vi "Autonomous Independent.vi"() -> ()   [LabVIEW 2020]
doc: "This VI is called when autonomous begins, and will automatically be terminated when autonomous ends. You can carry out timed or sensor driven robot movement independently without needing to return to the caller."
uses:
  <vilib>/Rock Robotics/WPI/Solenoid/WPI_SolenoidValue.ctl
  <vilib>/Rock Robotics/WPI/ThirdParty/Phoenix-LabVIEW/Motor Controller/Controls/CTRE_Phoenix_MotorControl_ControlMode.ctl
  <vilib>/Rock Robotics/WPI/Utilities/WPI_GetSetVariantRefNum.vi
  <vilib>/Rock Robotics/WPI/Solenoid/WPI_SolenoidSetEnum.vi
  <vilib>/Rock Robotics/Network Tables/NT Read Number.vi
  GlobalDriveJoysticks.vi
  <vilib>/Rock Robotics/Network Tables/NT Read String.vi
  <vilib>/Rock Robotics/Network Tables/NT Write Numeric Array.vi
panel:
  out "Orange Limit Pressed 8":bool
  out "Blue Limit Pressed 8":bool
  out "Ty 8":dbl
  out "Orange Limit Pressed 7":bool
  out "Blue Limit Pressed 7":bool
  out "Ty 7":dbl
  out "Intake 4":bool
  out "Elevate 4":bool
  out "Orange Limit Pressed 6":bool
  out "Blue Limit Pressed 6":bool
  out "Ty 6":dbl
  out "Orange Limit Pressed 5":bool
  out "Blue Limit Pressed 5":bool
  out "Ty 5":dbl
  out "Intake 3":bool
  out "Elevate 3":bool
  out "Orange Limit Pressed 4":bool
  out "Blue Limit Pressed 4":bool
  out "Ty 4":dbl
  out "Orange Limit Pressed 3":bool
  out "Blue Limit Pressed 3":bool
  out "Ty 3":dbl
  out "Intake 2":bool
  out "Elevate 2":bool
  out "Orange Limit Pressed 2":bool
  out "Blue Limit Pressed 2":bool
  out "Ty 2":dbl
  out "Ty":dbl
  out "Blue Limit Pressed":bool
  out "Orange Limit Pressed":bool
  out "Elevate":bool
  out "Intake":bool
  # "Be sure to right-click and choose Data Operations>>Make Current Value default if you want to save the array values with the VI"
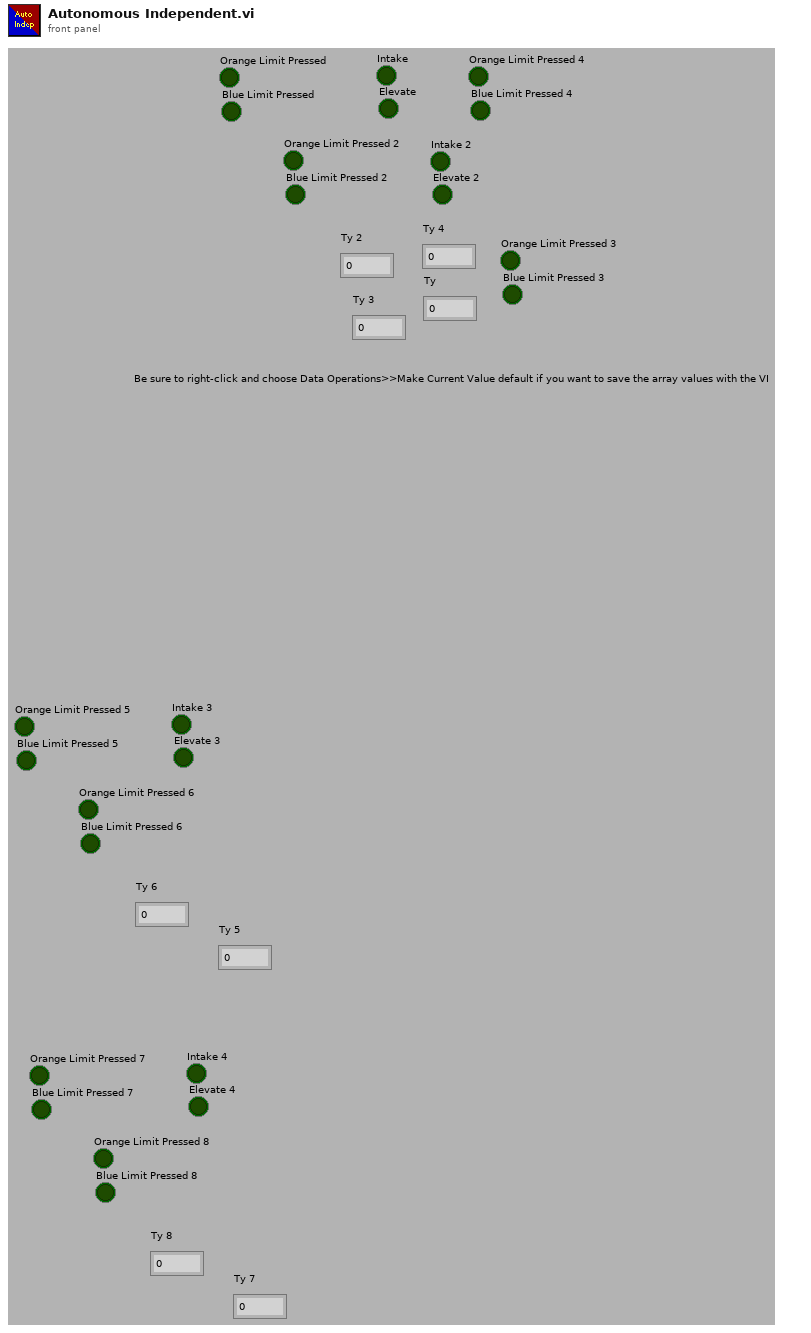
[diagram p1: front panel]
types:
  T1 = typedef "WPI_JoystickDevRef.ctl" = cluster{"Device":T2}
  T2 = typedef "WPI_JoystickDeviceEnum.ctl" = enum16{"USB 0", "USB 1", "USB 2", "USB 3", "USB 4", "USB 5"}
  T3 = typedef "WPI_SolenoidValue.ctl" = enum16{"Off", "On", "Forward", "Reverse"}
  T4 = typedef "WPI_SwitchDevRef.ctl" = cluster{"DevStatus":errorcluster, "DIO Channel":T5, "CntIndex":T6, "Normally Closed":bool}
  T5 = typedef "FPGA_DIOChannel.ctl" = enum8{"DIO 0", "DIO 1", "DIO 2", "DIO 3", "DIO 4", "DIO 5", "DIO 6", "DIO 7", "DIO 8", "DIO 9", "DIO MXP 0", "DIO MXP 1", "DIO MXP 2", "DIO MXP 3", "DIO MXP 4", "DIO MXP 5", "DIO MXP 6", "DIO MXP 7", "DIO MXP 8", "DIO MXP 9", "DIO MXP 10", "DIO MXP 11", "DIO MXP 12", "DIO MXP 13", "DIO MXP 14", "DIO MXP 15", "SPI Port CS1", "SPI Port CS2", "SPI Port CS3", "SPI Port MISO", "SPI Port MOSI", "Invalid"}
  T6 = typedef "FPGA_CounterCtrSystemIndex.ctl" = enum8{"Ctr 0", "Ctr 1", "Ctr 2", "Ctr 3", "Ctr 4", "Ctr 5", "Ctr 6", "Ctr 7", "Invalid"}
  T7 = typedef "WPI_SolenoidDevRef.ctl" = cluster{"DevStatus":errorcluster, "Pneumatics Control Module":u8, "Forward Solenoid Channel":T8, "Reverse Solenoid Channel":T8}
  T8 = typedef "WPI_SolenoidChannel.ctl" = enum8{"Solenoid 0", "Solenoid 1", "Solenoid 2", "Solenoid 3", "Solenoid 4", "Solenoid 5", "Solenoid 6", "Solenoid 7", "Solenoid 8", "Solenoid 9", "Solenoid 10", "Solenoid 11", "Solenoid 12", "Solenoid 13", "Solenoid 14", "Solenoid 15", "Invalid"}
  T9 = typedef "WPI_MotorControlDeviceRef.ctl" = cluster{"DeviceStatus":errorcluster, "Type":T10, "PWM":cluster{"PWM Channel":T11, "DeadBand":T12}, "CAN":cluster{"Device Number":u8, "SetOutput VI Ref":variant, "GetOutput VI Ref":variant, "Enable VI Ref":variant, "Disable VI Ref":variant, "Data":variant}, "Invert":bool, "DIO PWM":cluster{"PWM \"Enable\" Channel":T11, "DIOChannel":T5, "PWM Rate":dbl}}
  T10 = typedef "WPI_MotorControlType.ctl" = enum16{"PWM", "CAN", "DIO PWM"}
  T11 = typedef "FPGA_DIOPWMChannel.ctl" = enum8{"PWM 0", "PWM 1", "PWM 2", "PWM 3", "PWM 4", "PWM 5", "PWM 6", "PWM 7", "PWM 8", "PWM 9", "PWM MXP 0", "PWM MXP 1", "PWM MXP 2", "PWM MXP 3", "PWM MXP 4", "PWM MXP 5", "PWM MXP 6", "PWM MXP 7", "PWM MXP 8", "PWM MXP 9", "Invalid"}
  T12 = typedef "WPI_PWMDeadband.ctl" = cluster{"Name":string, "maxPositivePwm":i32, "minPositivePwm":i32, "centerPwm":i32, "maxNegativePwm":i32, "minNegativePwm":i32, "angularRange":u16}
  T13 = typedef "CTRE_Phoenix_MotorControl_ControlMode.ctl" = u16
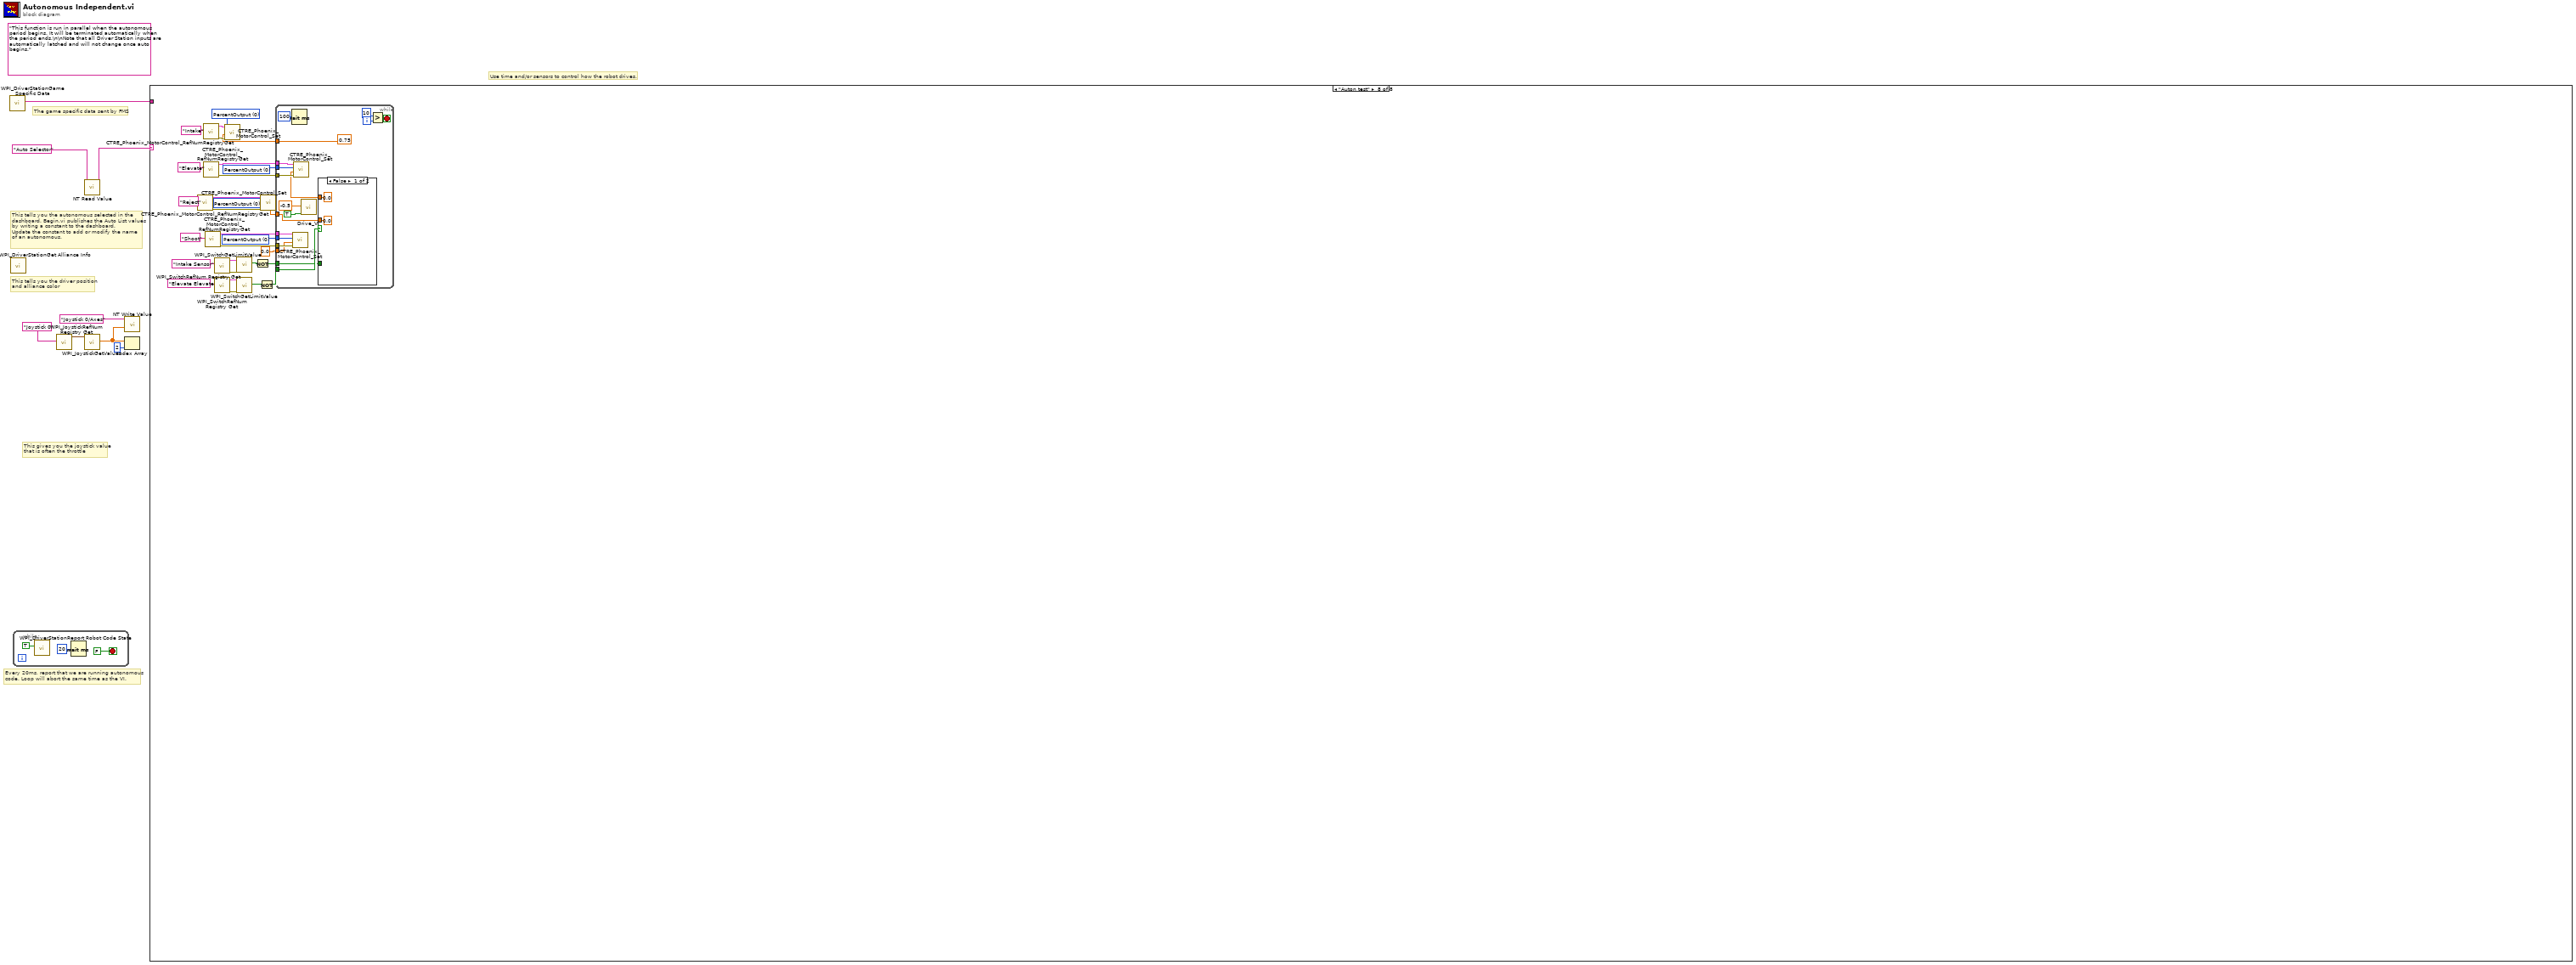
[diagram p0: block diagram]
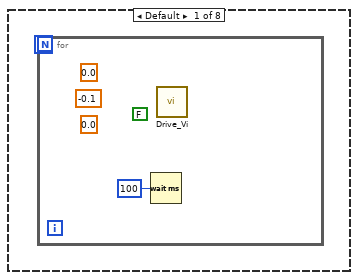
[diagram p2: hidden frame]
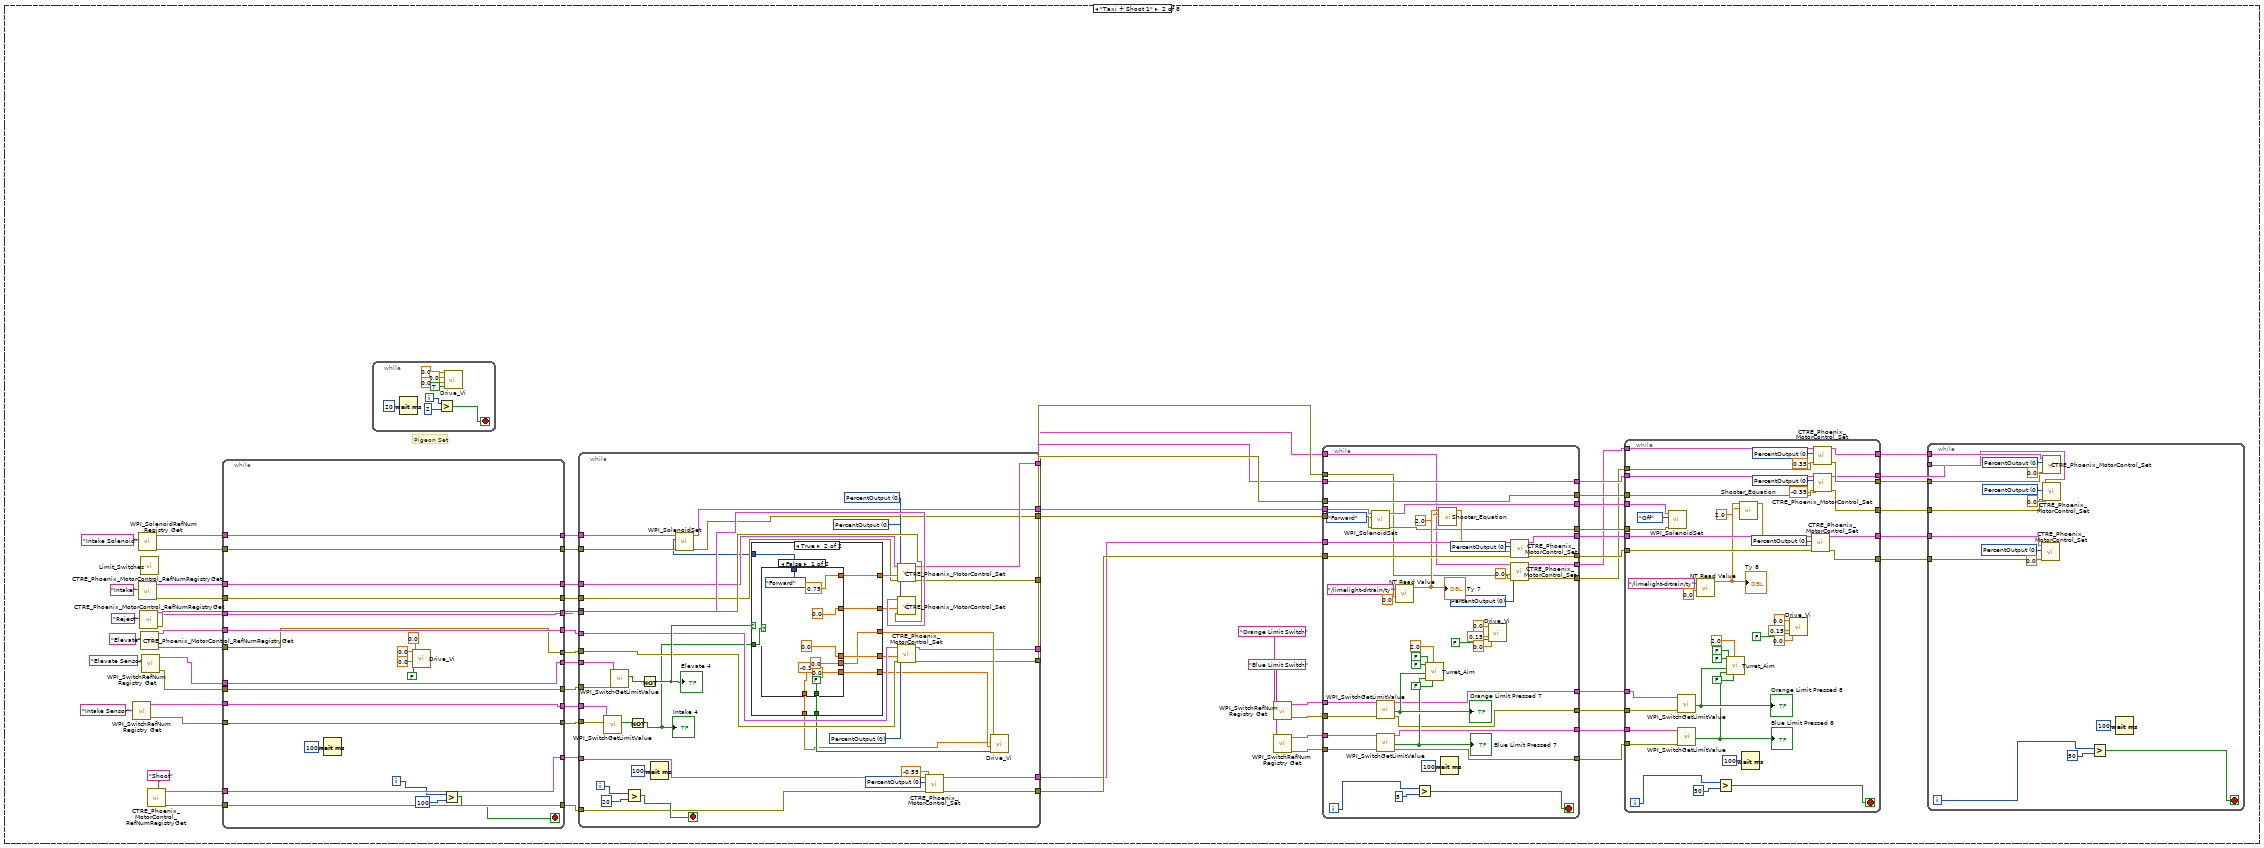
[diagram p3: hidden frame]
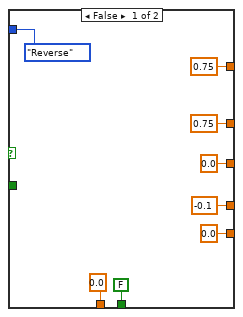
[diagram p4: hidden frame]
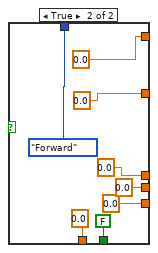
[diagram p5: hidden frame]
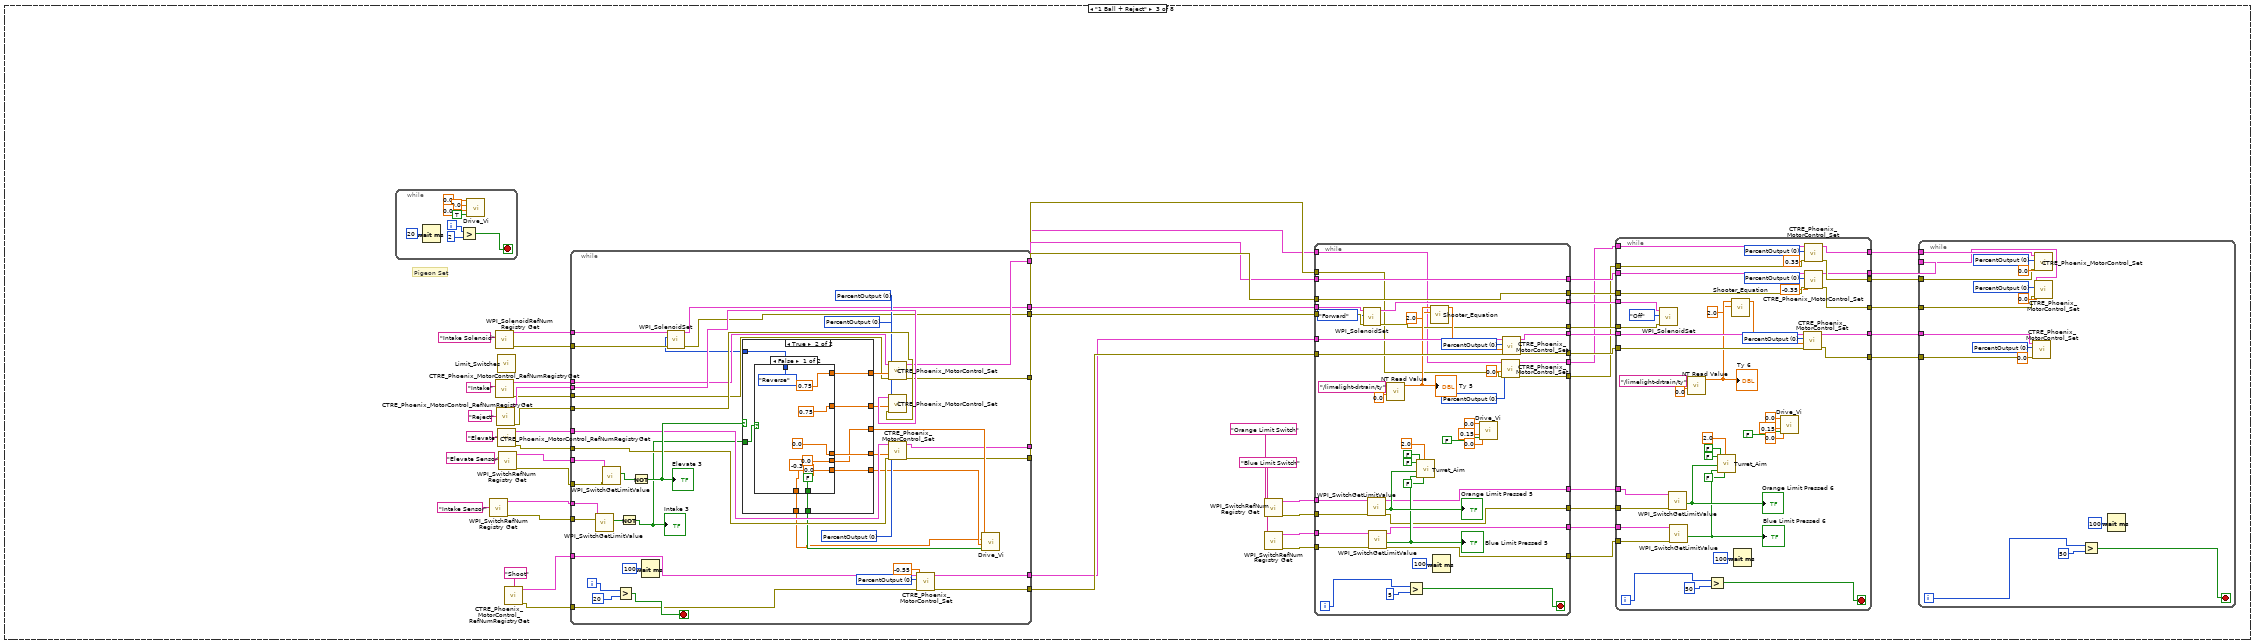
[diagram p6: hidden frame]
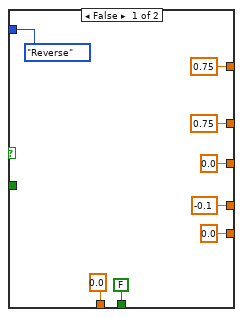
[diagram p7: hidden frame]
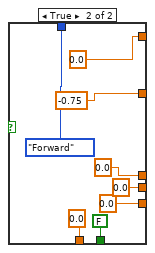
[diagram p8: hidden frame]
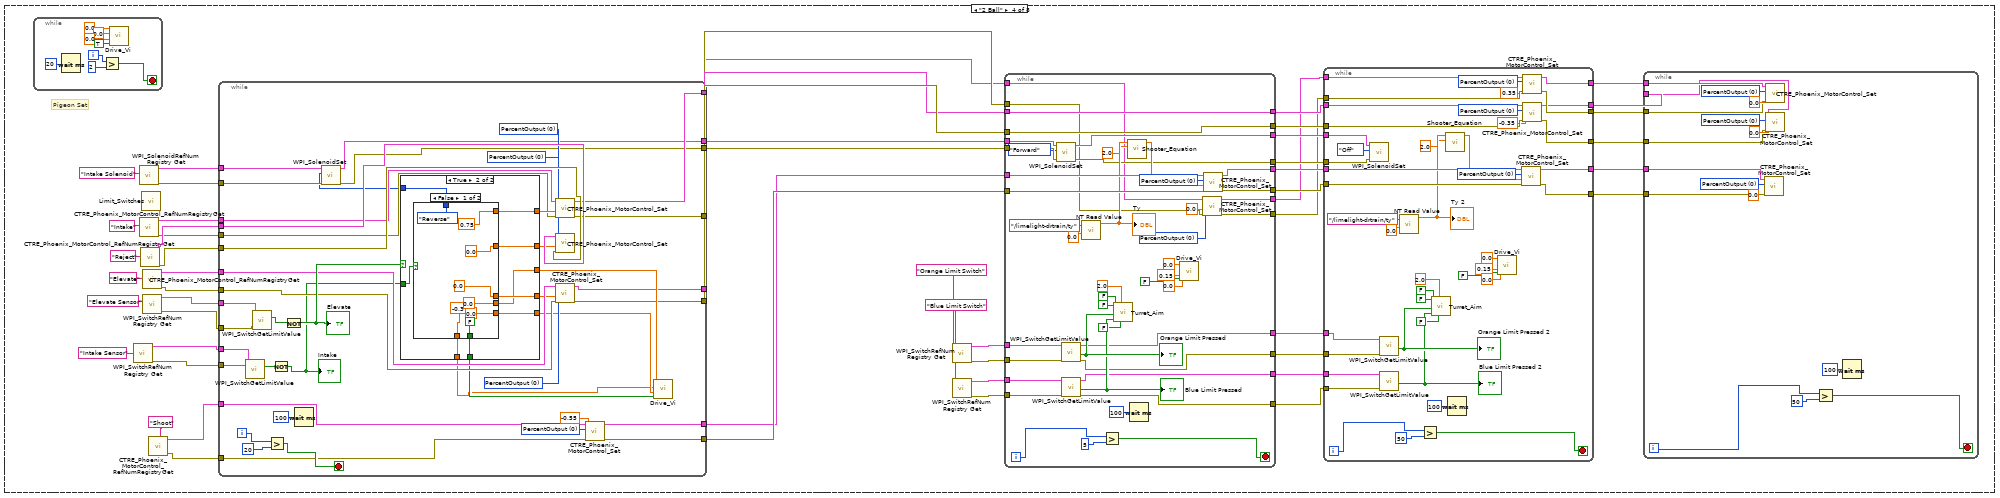
[diagram p9: hidden frame]
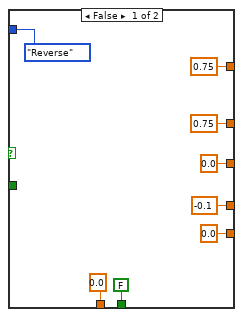
[diagram p10: hidden frame]
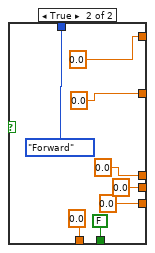
[diagram p11: hidden frame]
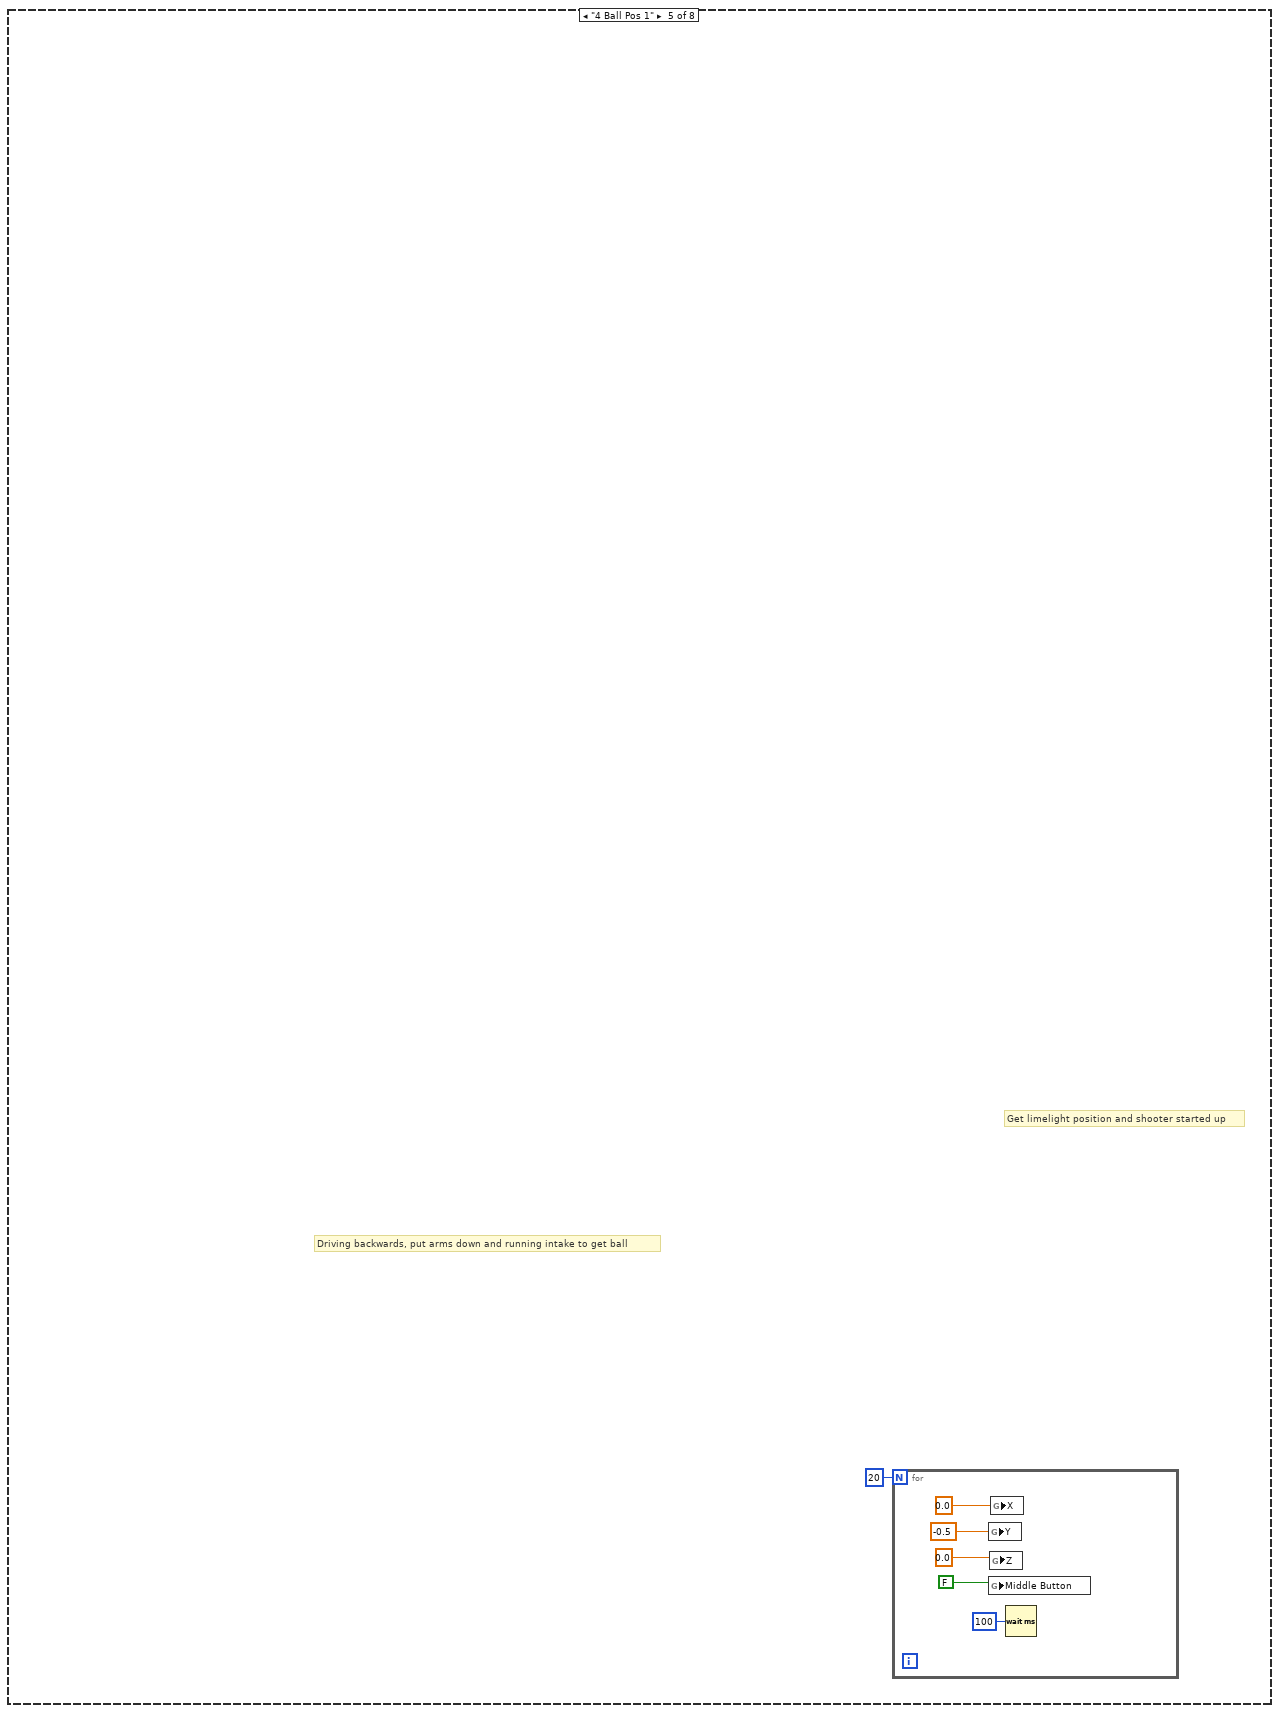
[diagram p12: hidden frame]
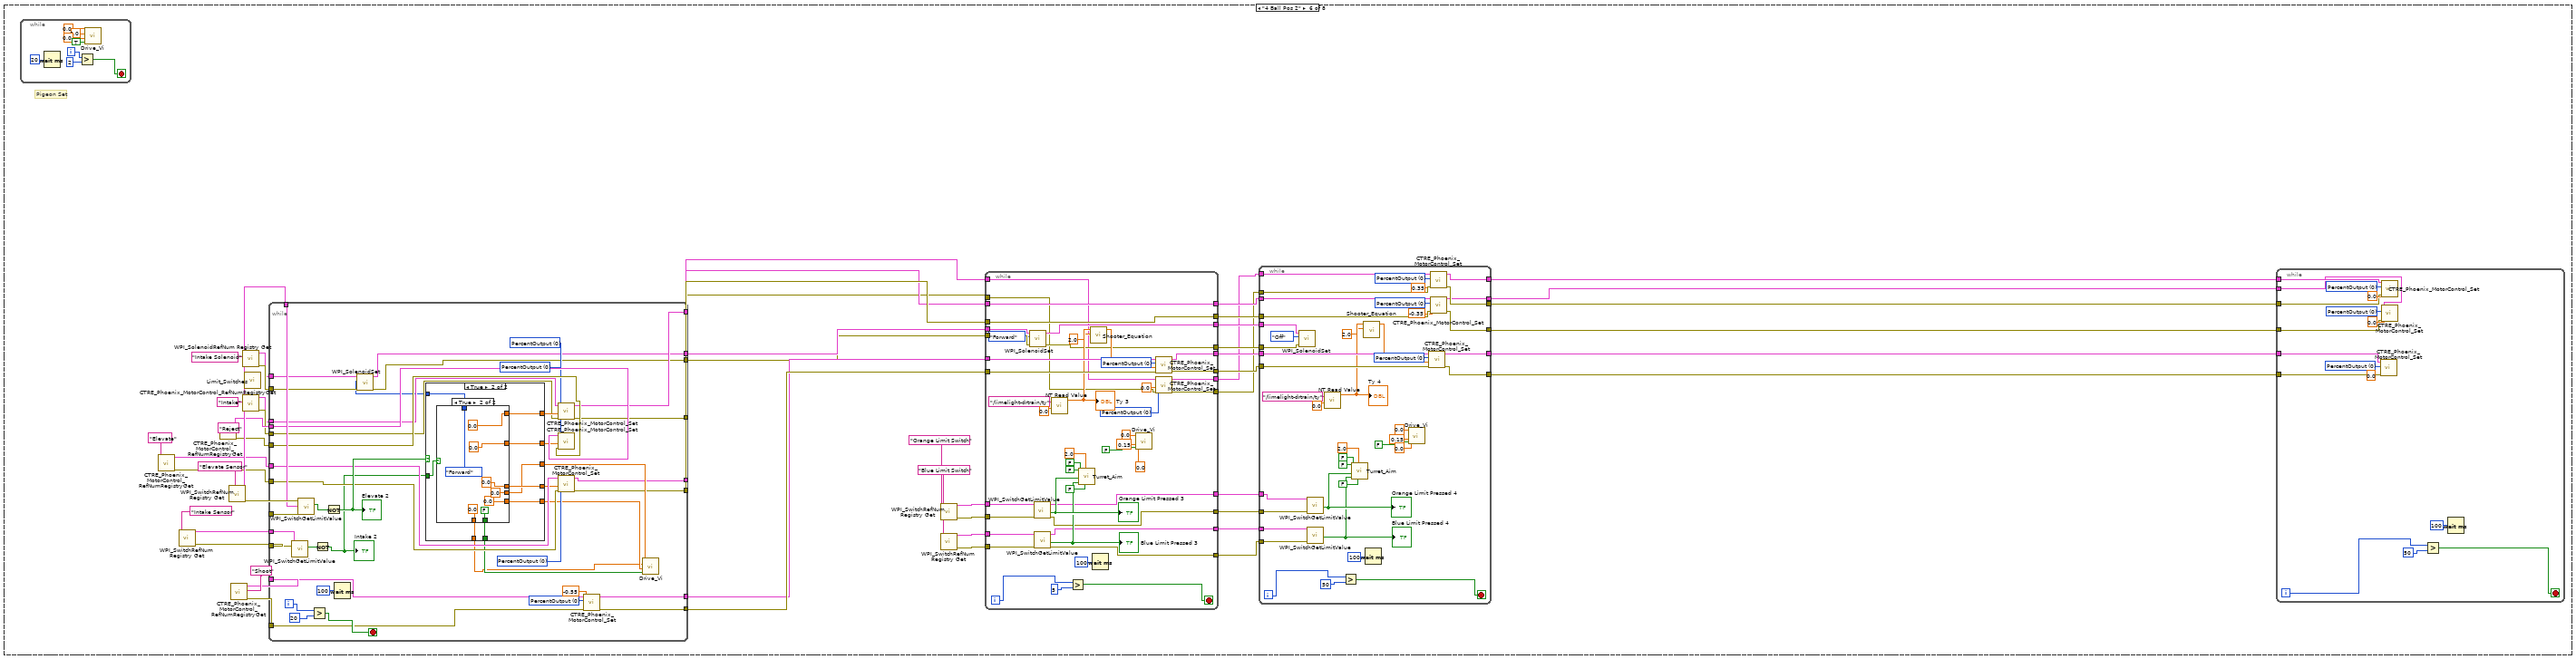
[diagram p13: hidden frame]
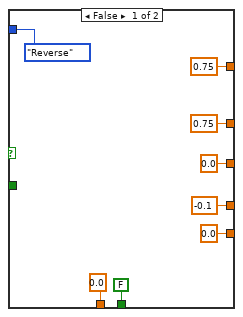
[diagram p14: hidden frame]
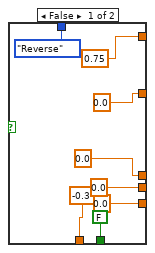
[diagram p15: hidden frame]
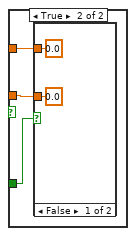
[diagram p17: hidden frame]
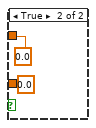
[diagram p18: hidden frame]
diagram:
  (unwired) "This function is run in parallel when the autonomous period begins. It will be terminated automatically when the period ends.\n\nNote that all Driver Station inputs are automatically latched and will not change once auto begins."
  # "The game specific data sent by FMS"
  # "This tells you the autonomous selected in the \ndashboard. Begin.vi publishes the Auto List values\nby writing a constant to the dashboard.\nUpdate the constant to add or modify the name\nof an autonomous."
  # "Every 20ms, report that we are running autonomous\ncode. Loop will abort the same time as the VI."
  # "This gives you the joystick value\nthat is often the throttle"
  # "Use time and/or sensors to control how the robot drives."
  # "This tells you the driver position\nand alliance color"
  n1 = call <vilib>:"WPI_DriverStationGame Specific Data.vi"() -> ("Game Specific Data"=w1:string)  [unwired: 11 in]
  n2 = call <vilib>:"WPI_DriverStationGet Alliance Info.vi"() -> ()  [unwired: 12 out]
  n3 = while {
    stop <- FALSE stop-if-true
    n4 = call <vilib>:"WPI_DriverStationReport Robot Code State.vi"("Autonomous"=TRUE) -> ()  [unwired: 10 in, 1 out]
    n5 = Wait (ms)(milliseconds to wait=u32 20) -> ()  [unwired: 1 out]
  }
  n6 = call <vilib>:"WPI_JoystickRefNum Registry Get.vi"("refnum name"="Joystick 0") -> ("JoystickDevRef"=w7:T1)  [unwired: 1 in, 9 out]
  n7 = call <vilib>:"WPI_JoystickGetValues.vi"("JoystickDevRef"=w7) -> ("Axes"=w3:dbl[])  [unwired: 6 in, 4 out]
  n8 = call-poly <vilib>:"NT Read Value.vi"("Name"="Auto Selector") -> ("String"=w4:string)  [unwired: 9 in, 1 out]
  n9 = call-poly <vilib>:"NT Write Value.vi"("Numeric Array"=w3, "Name"="Joystick 0/Axes") -> ()  [unwired: 9 in, 1 out]
  n10 = Index Array(array=w3, index=2) -> ()  [unwired: 1 out]
  n11 = case shown="\"Auton test\"" w4 {
    tunnel: w1 -> [_ _ _ _ _ _ _ _]
    frame Default {
      n12 = for {
        N: 20 -> [_]
        (unwired) FALSE ("Middle Thumb")
        (unwired) 0.0 ("Z")
        (unwired) -0.1 ("Y")
        (unwired) 0.0 ("X")
        n13 = Wait (ms)(milliseconds to wait=u32 100) -> ()  [unwired: 1 out]
        n14 = call "Drive_Vi.vi"() -> ()  [unwired: 12 in]
      }
    }
    frame "Taxi + Shoot 1" {
      # "Pigeon Set"
      n15 = call <vilib>:"WPI_SwitchRefNum Registry Get.vi"("refnum name"="Intake Sensor") -> ("error out"=w18:errorcluster, "SwitchDevRef"=w20:T4)  [unwired: 9 in]
      n16 = call <vilib>:"WPI_SolenoidRefNum Registry Get.vi"("refnum name"="Intake Solenoid") -> ("error out"=w37:errorcluster, "SolenoidDevRef"=w39:T7)  [unwired: 9 in]
      n17 = call <vilib>:"CTRE_Phoenix_MotorControl_RefNumRegistryGet.vi"("refnum name"="Intake") -> ("error out"=w32:errorcluster, "PhoenixMotorControlDevRef"=w34:T9)  [unwired: 9 in]
      n18 = call <vilib>:"CTRE_Phoenix_MotorControl_RefNumRegistryGet.vi"("refnum name"="Reject") -> ("error out"=w72:errorcluster, "PhoenixMotorControlDevRef"=w30:T9)  [unwired: 9 in]
      n19 = call "Limit_Switches.vi"() -> ()  [unwired: 10 in, 2 out]
      n20 = call <vilib>:"CTRE_Phoenix_MotorControl_RefNumRegistryGet.vi"("refnum name"="Elevate") -> ("error out"=w26:errorcluster, "PhoenixMotorControlDevRef"=w28:T9)  [unwired: 9 in]
      n21 = call <vilib>:"WPI_SwitchRefNum Registry Get.vi"("refnum name"="Elevate Sensor") -> ("error out"=w22:errorcluster, "SwitchDevRef"=w24:T4)  [unwired: 9 in]
      n22 = call <vilib>:"CTRE_Phoenix_MotorControl_RefNumRegistryGet.vi"("refnum name"="Shoot") -> ("error out"=w14:errorcluster, "PhoenixMotorControlDevRef"=w17:T9)  [unwired: 9 in]
      n23 = while {
        tunnel: [w96] -> w38
        tunnel: w39 -> [w96]
        tunnel: [w95] -> w36
        tunnel: w37 -> [w95]
        tunnel: [w94] -> w35
        tunnel: w34 -> [w94]
        tunnel: [w93] -> w33
        tunnel: w32 -> [w93]
        tunnel: [w92] -> w31
        tunnel: w30 -> [w92]
        tunnel: [w91] -> w29
        tunnel: w28 -> [w91]
        tunnel: [w90] -> w27
        tunnel: w26 -> [w90]
        tunnel: [w89] -> w25
        tunnel: w24 -> [w89]
        tunnel: [w88] -> w23
        tunnel: w22 -> [w88]
        tunnel: [w87] -> w21
        tunnel: w20 -> [w87]
        tunnel: [w86] -> w19
        tunnel: w18 -> [w86]
        tunnel: [w85] -> w16
        tunnel: w17 -> [w85]
        tunnel: [w84] -> w15
        tunnel: w14 -> [w84]
        i -> [w80]
        stop <- w82 stop-if-true
        n24 = Wait (ms)(milliseconds to wait=u32 100) -> ()  [unwired: 1 out]
        n25 = call "Drive_Vi.vi"("Middle Thumb"=FALSE, "Z"=0.0, "Y"=0.0, "X"=0.0) -> ()  [unwired: 8 in]
        n26 = Greater?(x=w80, y=100) -> (0:w82:bool)
      }
      n27 = while {
        i -> [w286]
        stop <- w287 stop-if-true
        n28 = Wait (ms)(milliseconds to wait=u32 20) -> ()  [unwired: 1 out]
        n29 = Greater?(x=w286, y=2) -> (0:w287:bool)
        n30 = call "Drive_Vi.vi"("Middle Thumb"=TRUE, "Z"=0.0, "Y"=0.0, "X"=0.0) -> ()  [unwired: 8 in]
      }
      n31 = while {
        tunnel: w23 -> [w241]
        tunnel: w25 -> [w240]
        tunnel: w19 -> [w239]
        tunnel: w21 -> [w238]
        tunnel: w36 -> [w237]
        tunnel: w38 -> [w236]
        tunnel: w27 -> [w233]
        tunnel: w29 -> [w232]
        tunnel: w72 -> [w231]
        tunnel: w31 -> [w230]
        tunnel: w33 -> [w229]
        tunnel: w35 -> [w228]
        tunnel: [w216] -> w65
        tunnel: [w215] -> w64
        tunnel: [w214] -> w63
        tunnel: [w213] -> w62
        tunnel: w15 -> [w212]
        tunnel: w16 -> [w211]
        tunnel: [w208] -> w61
        tunnel: [w207] -> w60
        tunnel: [w206] -> w51
        tunnel: [w205] -> w50
        i -> [w244]
        stop <- w245 stop-if-true
        w210 = T13 0 items=["PercentOutput"=0, "Position"=1, "Velocity"=2, "Current"=3, "Follower"=5, "MotionProfile"=6, "MotionMagic"=7, "MotionProfileArc"=10, "Disabled"=15] ("Control Mode")
        w222 = T13 0 items=["PercentOutput"=0, "Position"=1, "Velocity"=2, "Current"=3, "Follower"=5, "MotionProfile"=6, "MotionMagic"=7, "MotionProfileArc"=10, "Disabled"=15] ("Control Mode")
        w223 = T13 0 items=["PercentOutput"=0, "Position"=1, "Velocity"=2, "Current"=3, "Follower"=5, "MotionProfile"=6, "MotionMagic"=7, "MotionProfileArc"=10, "Disabled"=15] ("Control Mode")
        w224 = T13 0 items=["PercentOutput"=0, "Position"=1, "Velocity"=2, "Current"=3, "Follower"=5, "MotionProfile"=6, "MotionMagic"=7, "MotionProfileArc"=10, "Disabled"=15] ("Control Mode")
        n32 = call <vilib>:"WPI_SwitchGetLimitValue.vi"("error in (no error)"=w239, "SwitchDevRef"=w238) -> ("Switch Pressed"=w242:bool)  [unwired: 7 in, 2 out]
        n33 = call <vilib>:"WPI_SwitchGetLimitValue.vi"("error in (no error)"=w241, "SwitchDevRef"=w240) -> ("Switch Pressed"=w243:bool)  [unwired: 7 in, 2 out]
        n34 = Greater?(x=w244, y=20) -> (0:w245:bool)
        n35 = Not(x=w242) -> (.not. x?=w227:bool)
        "Intake 4" <- w227
        n36 = Not(x=w243) -> (.not. x?=w235:bool)
        "Elevate 4" <- w235
        n37 = Wait (ms)(milliseconds to wait=u32 100) -> ()  [unwired: 1 out]
        n38 = case shown="True" w235 {
          tunnel: [0.75 ("Output") w264] -> w234
          tunnel: w227 -> [_ w261]
          tunnel: [0.75 ("Output") w263] -> w226
          tunnel: [-0.1 ("Output") w262] -> w225
          tunnel: [FALSE ("Middle Thumb") w260] -> w221
          tunnel: [0.0 ("Z") w259] -> w220
          tunnel: [0.0 ("Y") w258] -> w219
          tunnel: [0.0 ("X") w257] -> w218
          tunnel: [WPI_SolenoidValue."Reverse" ("Value") w256] -> w217
          frame False {
          }
          frame True {
            n39 = case shown="False" w261 {
              tunnel: [0.75 ("Output") 0.0 ("Output")] -> w264
              tunnel: [0.0 ("Output") 0.0 ("Output")] -> w263
              tunnel: [0.0 ("Output") 0.0 ("Output")] -> w262
              tunnel: [FALSE ("Middle Thumb") FALSE ("Middle Thumb")] -> w260
              tunnel: [0.0 ("Z") 0.0 ("Z")] -> w259
              tunnel: [-0.3 ("Y") 0.0 ("Y")] -> w258
              tunnel: [0.0 ("X") 0.0 ("X")] -> w257
              tunnel: [WPI_SolenoidValue."Forward" ("Value") WPI_SolenoidValue."Forward" ("Value")] -> w256
              frame False {
              }
              frame True {
              }
            }
          }
        }
        n40 = call-poly <vilib>:"WPI_SolenoidSet.vi"("error in (no error)"=w237, "Value"=w217, "SolenoidDevRef"=w236) -> ("error out"=w205:errorcluster, "SolenoidDevRef"=w206:T7)  [unwired: 7 in]
        n41 = call <vilib>:"CTRE_Phoenix_MotorControl_Set.vi"("error in (no error)"=w229, "Output"=w234, "Control Mode"=w222, "PhoenixMotorControlDevRef"=w228) -> ("error out"=w214:errorcluster, "PhoenixMotorControlDevRef"=w213:T9)  [unwired: 6 in]
        n42 = call <vilib>:"CTRE_Phoenix_MotorControl_Set.vi"("error in (no error)"=w231, "Output"=w226, "Control Mode"=w223, "PhoenixMotorControlDevRef"=w230) -> ()  [unwired: 6 in, 2 out]
        n43 = call <vilib>:"CTRE_Phoenix_MotorControl_Set.vi"("error in (no error)"=w233, "Output"=w225, "Control Mode"=w224, "PhoenixMotorControlDevRef"=w232) -> ("error out"=w216:errorcluster, "PhoenixMotorControlDevRef"=w215:T9)  [unwired: 6 in]
        n44 = call <vilib>:"CTRE_Phoenix_MotorControl_Set.vi"("error in (no error)"=w212, "Output"=-0.55, "Control Mode"=w210, "PhoenixMotorControlDevRef"=w211) -> ("error out"=w208:errorcluster, "PhoenixMotorControlDevRef"=w207:T9)  [unwired: 6 in]
        n45 = call "Drive_Vi.vi"("Middle Thumb"=w221, "Z"=w220, "Y"=w219, "X"=w218) -> ()  [unwired: 8 in]
      }
      n46 = call <vilib>:"WPI_SwitchRefNum Registry Get.vi"("refnum name"="Orange Limit Switch") -> ("error out"=w67:errorcluster, "SwitchDevRef"=w66:T4)  [unwired: 9 in]
      n47 = call <vilib>:"WPI_SwitchRefNum Registry Get.vi"("refnum name"="Blue Limit Switch") -> ("error out"=w69:errorcluster, "SwitchDevRef"=w68:T4)  [unwired: 9 in]
      n48 = while {
        tunnel: w61 -> [w204]
        tunnel: w60 -> [w203]
        tunnel: w69 -> [w200]
        tunnel: w68 -> [w199]
        tunnel: w67 -> [w198]
        tunnel: w66 -> [w197]
        tunnel: w65 -> [w172]
        tunnel: w64 -> [w171]
        tunnel: w63 -> [w162]
        tunnel: w62 -> [w163]
        tunnel: [w178] -> w59
        tunnel: [w177] -> w58
        tunnel: [w176] -> w57
        tunnel: [w175] -> w56
        tunnel: [w174] -> w55
        tunnel: [w173] -> w54
        tunnel: [w172] -> w53
        tunnel: [w171] -> w52
        tunnel: w51 -> [w170]
        tunnel: w50 -> [w169]
        tunnel: [w167] -> w49
        tunnel: [w166] -> w48
        tunnel: [w165] -> w47
        tunnel: [w164] -> w46
        i -> [w185]
        stop <- w183 stop-if-true
        w161 = T13 0 items=["PercentOutput"=0, "Position"=1, "Velocity"=2, "Current"=3, "Follower"=5, "MotionProfile"=6, "MotionMagic"=7, "MotionProfileArc"=10, "Disabled"=15] ("Control Mode")
        w184 = T13 0 items=["PercentOutput"=0, "Position"=1, "Velocity"=2, "Current"=3, "Follower"=5, "MotionProfile"=6, "MotionMagic"=7, "MotionProfileArc"=10, "Disabled"=15] ("Control Mode")
        n49 = call-poly <vilib>:"WPI_SolenoidSet.vi"("error in (no error)"=w169, "Value"=WPI_SolenoidValue."Forward", "SolenoidDevRef"=w170) -> ("error out"=w166:errorcluster, "SolenoidDevRef"=w167:T7)  [unwired: 7 in]
        n50 = call <vilib>:"WPI_SwitchGetLimitValue.vi"("error in (no error)"=w198, "SwitchDevRef"=w197) -> ("error out"=w175:errorcluster, "Switch Pressed"=w196:bool, "SwitchDevRef"=w176:T4)  [unwired: 7 in]
        "Orange Limit Pressed 7" <- w196
        n51 = call <vilib>:"WPI_SwitchGetLimitValue.vi"("error in (no error)"=w200, "SwitchDevRef"=w199) -> ("error out"=w177:errorcluster, "Switch Pressed"=w195:bool, "SwitchDevRef"=w178:T4)  [unwired: 7 in]
        "Blue Limit Pressed 7" <- w195
        n52 = call-poly <vilib>:"NT Read Value.vi"("Default Value"=0.0, "Name"="/limelight-drtrain/ty") -> ("Numeric"=w189:dbl)  [unwired: 8 in, 1 out]
        "Ty 7" <- w189
        n53 = Greater?(x=w185, y=5) -> (0:w183:bool)
        n54 = call "Turret_Aim.vi"("View Button"=FALSE ("Driver Right Thumb"), "Left Trigger"=2.0, "Orange Limit Pressed"=w195, "Blue Limit Pressed"=w196, "Right Bumper"=FALSE, "Left Bumper"=FALSE) -> ()  [unwired: 6 in]
        n55 = call "Shooter_Equation.vi"("Right Trigger"=2.0, "Ty"=w189) -> ("% voltage"=w192:dbl)  [unwired: 9 in]
        n56 = Wait (ms)(milliseconds to wait=u32 100) -> ()  [unwired: 1 out]
        n57 = call "Drive_Vi.vi"("Middle Thumb"=FALSE, "Z"=0.0, "Y"=0.15, "X"=0.0) -> ()  [unwired: 8 in]
        n58 = call <vilib>:"CTRE_Phoenix_MotorControl_Set.vi"("error in (no error)"=w162, "Output"=0.0, "Control Mode"=w161, "PhoenixMotorControlDevRef"=w163) -> ("error out"=w164:errorcluster, "PhoenixMotorControlDevRef"=w165:T9)  [unwired: 6 in]
        n59 = call <vilib>:"CTRE_Phoenix_MotorControl_Set.vi"("error in (no error)"=w204, "Output"=w192, "Control Mode"=w184, "PhoenixMotorControlDevRef"=w203) -> ("error out"=w174:errorcluster, "PhoenixMotorControlDevRef"=w173:T9)  [unwired: 6 in]
      }
      n60 = while {
        tunnel: w55 -> [w159]
        tunnel: w54 -> [w158]
        tunnel: w58 -> [w155]
        tunnel: w59 -> [w154]
        tunnel: w56 -> [w153]
        tunnel: w53 -> [w138]
        tunnel: w52 -> [w137]
        tunnel: w46 -> [w136]
        tunnel: w47 -> [w135]
        tunnel: w57 -> [w126]
        tunnel: w49 -> [w125]
        tunnel: w48 -> [w124]
        tunnel: [w122] -> w45
        tunnel: [w121] -> w44
        tunnel: [w120] -> w43
        tunnel: [w119] -> w42
        tunnel: [w118] -> w41
        tunnel: [w117] -> w40
        i -> [w141]
        stop <- w139 stop-if-true
        w133 = T13 0 items=["PercentOutput"=0, "Position"=1, "Velocity"=2, "Current"=3, "Follower"=5, "MotionProfile"=6, "MotionMagic"=7, "MotionProfileArc"=10, "Disabled"=15] ("Control Mode")
        w134 = T13 0 items=["PercentOutput"=0, "Position"=1, "Velocity"=2, "Current"=3, "Follower"=5, "MotionProfile"=6, "MotionMagic"=7, "MotionProfileArc"=10, "Disabled"=15] ("Control Mode")
        w140 = T13 0 items=["PercentOutput"=0, "Position"=1, "Velocity"=2, "Current"=3, "Follower"=5, "MotionProfile"=6, "MotionMagic"=7, "MotionProfileArc"=10, "Disabled"=15] ("Control Mode")
        n61 = call-poly <vilib>:"WPI_SolenoidSet.vi"("error in (no error)"=w124, "Value"=WPI_SolenoidValue."Off", "SolenoidDevRef"=w125) -> ()  [unwired: 7 in, 2 out]
        n62 = call <vilib>:"WPI_SwitchGetLimitValue.vi"("error in (no error)"=w153, "SwitchDevRef"=w126) -> ("Switch Pressed"=w152:bool)  [unwired: 7 in, 2 out]
        "Orange Limit Pressed 8" <- w152
        n63 = call <vilib>:"WPI_SwitchGetLimitValue.vi"("error in (no error)"=w155, "SwitchDevRef"=w154) -> ("Switch Pressed"=w151:bool)  [unwired: 7 in, 2 out]
        "Blue Limit Pressed 8" <- w151
        n64 = call-poly <vilib>:"NT Read Value.vi"("Default Value"=0.0, "Name"="/limelight-drtrain/ty") -> ("Numeric"=w145:dbl)  [unwired: 8 in, 1 out]
        "Ty 8" <- w145
        n65 = Greater?(x=w141, y=50) -> (0:w139:bool)
        n66 = call "Turret_Aim.vi"("View Button"=FALSE ("Driver Right Thumb"), "Left Trigger"=2.0, "Orange Limit Pressed"=w151, "Blue Limit Pressed"=w152, "Right Bumper"=FALSE, "Left Bumper"=FALSE) -> ()  [unwired: 6 in]
        n67 = call "Shooter_Equation.vi"("Right Trigger"=2.0, "Ty"=w145) -> ("% voltage"=w148:dbl)  [unwired: 9 in]
        n68 = Wait (ms)(milliseconds to wait=u32 100) -> ()  [unwired: 1 out]
        n69 = call "Drive_Vi.vi"("Middle Thumb"=FALSE, "Z"=0.0, "Y"=0.15, "X"=0.0) -> ()  [unwired: 8 in]
        n70 = call <vilib>:"CTRE_Phoenix_MotorControl_Set.vi"("error in (no error)"=w159, "Output"=w148, "Control Mode"=w140, "PhoenixMotorControlDevRef"=w158) -> ("error out"=w117:errorcluster, "PhoenixMotorControlDevRef"=w118:T9)  [unwired: 6 in]
        n71 = call <vilib>:"CTRE_Phoenix_MotorControl_Set.vi"("error in (no error)"=w136, "Output"=0.35, "Control Mode"=w133, "PhoenixMotorControlDevRef"=w135) -> ("error out"=w122:errorcluster, "PhoenixMotorControlDevRef"=w121:T9)  [unwired: 6 in]
        n72 = call <vilib>:"CTRE_Phoenix_MotorControl_Set.vi"("error in (no error)"=w138, "Output"=-0.35, "Control Mode"=w134, "PhoenixMotorControlDevRef"=w137) -> ("error out"=w119:errorcluster, "PhoenixMotorControlDevRef"=w120:T9)  [unwired: 6 in]
      }
      n73 = while {
        tunnel: w45 -> [w111]
        tunnel: w44 -> [w110]
        tunnel: w43 -> [w109]
        tunnel: w42 -> [w108]
        tunnel: w41 -> [w107]
        tunnel: w40 -> [w106]
        i -> [w103]
        stop <- w102 stop-if-true
        w114 = T13 0 items=["PercentOutput"=0, "Position"=1, "Velocity"=2, "Current"=3, "Follower"=5, "MotionProfile"=6, "MotionMagic"=7, "MotionProfileArc"=10, "Disabled"=15] ("Control Mode")
        w115 = T13 0 items=["PercentOutput"=0, "Position"=1, "Velocity"=2, "Current"=3, "Follower"=5, "MotionProfile"=6, "MotionMagic"=7, "MotionProfileArc"=10, "Disabled"=15] ("Control Mode")
        w116 = T13 0 items=["PercentOutput"=0, "Position"=1, "Velocity"=2, "Current"=3, "Follower"=5, "MotionProfile"=6, "MotionMagic"=7, "MotionProfileArc"=10, "Disabled"=15] ("Control Mode")
        n74 = call <vilib>:"CTRE_Phoenix_MotorControl_Set.vi"("error in (no error)"=w106, "Output"=0.0, "Control Mode"=w116, "PhoenixMotorControlDevRef"=w107) -> ()  [unwired: 6 in, 2 out]
        n75 = call <vilib>:"CTRE_Phoenix_MotorControl_Set.vi"("error in (no error)"=w111, "Output"=0.0, "Control Mode"=w114, "PhoenixMotorControlDevRef"=w110) -> ()  [unwired: 6 in, 2 out]
        n76 = call <vilib>:"CTRE_Phoenix_MotorControl_Set.vi"("error in (no error)"=w108, "Output"=0.0, "Control Mode"=w115, "PhoenixMotorControlDevRef"=w109) -> ()  [unwired: 6 in, 2 out]
        n77 = Greater?(x=w103, y=50) -> (0:w102:bool)
        n78 = Wait (ms)(milliseconds to wait=u32 100) -> ()  [unwired: 1 out]
      }
    }
    frame "1 Ball + Reject" {
      # "Pigeon Set"
      n79 = while {
        i -> [w527]
        stop <- w528 stop-if-true
        n80 = Wait (ms)(milliseconds to wait=u32 20) -> ()  [unwired: 1 out]
        n81 = Greater?(x=w527, y=2) -> (0:w528:bool)
        n82 = call "Drive_Vi.vi"("Middle Thumb"=TRUE, "Z"=0.0, "Y"=0.0, "X"=0.0) -> ()  [unwired: 8 in]
      }
      n83 = call <vilib>:"WPI_SwitchRefNum Registry Get.vi"("refnum name"="Intake Sensor") -> ("error out"=w332:errorcluster, "SwitchDevRef"=w331:T4)  [unwired: 9 in]
      n84 = call <vilib>:"WPI_SolenoidRefNum Registry Get.vi"("refnum name"="Intake Solenoid") -> ("error out"=w330:errorcluster, "SolenoidDevRef"=w329:T7)  [unwired: 9 in]
      n85 = call <vilib>:"CTRE_Phoenix_MotorControl_RefNumRegistryGet.vi"("refnum name"="Intake") -> ("error out"=w324:errorcluster, "PhoenixMotorControlDevRef"=w323:T9)  [unwired: 9 in]
      n86 = call <vilib>:"CTRE_Phoenix_MotorControl_RefNumRegistryGet.vi"("refnum name"="Reject") -> ("error out"=w326:errorcluster, "PhoenixMotorControlDevRef"=w325:T9)  [unwired: 9 in]
      n87 = call "Limit_Switches.vi"() -> ()  [unwired: 10 in, 2 out]
      n88 = call <vilib>:"CTRE_Phoenix_MotorControl_RefNumRegistryGet.vi"("refnum name"="Elevate") -> ("error out"=w328:errorcluster, "PhoenixMotorControlDevRef"=w327:T9)  [unwired: 9 in]
      n89 = call <vilib>:"WPI_SwitchRefNum Registry Get.vi"("refnum name"="Elevate Sensor") -> ("error out"=w334:errorcluster, "SwitchDevRef"=w333:T4)  [unwired: 9 in]
      n90 = call <vilib>:"CTRE_Phoenix_MotorControl_RefNumRegistryGet.vi"("refnum name"="Shoot") -> ("error out"=w312:errorcluster, "PhoenixMotorControlDevRef"=w311:T9)  [unwired: 9 in]
      n91 = while {
        tunnel: w334 -> [w482]
        tunnel: w333 -> [w481]
        tunnel: w332 -> [w480]
        tunnel: w331 -> [w479]
        tunnel: w330 -> [w478]
        tunnel: w329 -> [w477]
        tunnel: w328 -> [w474]
        tunnel: w327 -> [w473]
        tunnel: w326 -> [w472]
        tunnel: w325 -> [w471]
        tunnel: w324 -> [w470]
        tunnel: w323 -> [w469]
        tunnel: [w457] -> w316
        tunnel: [w456] -> w315
        tunnel: [w455] -> w314
        tunnel: [w454] -> w313
        tunnel: w312 -> [w453]
        tunnel: w311 -> [w452]
        tunnel: [w449] -> w310
        tunnel: [w448] -> w309
        tunnel: [w447] -> w300
        tunnel: [w446] -> w299
        i -> [w485]
        stop <- w486 stop-if-true
        w451 = T13 0 items=["PercentOutput"=0, "Position"=1, "Velocity"=2, "Current"=3, "Follower"=5, "MotionProfile"=6, "MotionMagic"=7, "MotionProfileArc"=10, "Disabled"=15] ("Control Mode")
        w463 = T13 0 items=["PercentOutput"=0, "Position"=1, "Velocity"=2, "Current"=3, "Follower"=5, "MotionProfile"=6, "MotionMagic"=7, "MotionProfileArc"=10, "Disabled"=15] ("Control Mode")
        w464 = T13 0 items=["PercentOutput"=0, "Position"=1, "Velocity"=2, "Current"=3, "Follower"=5, "MotionProfile"=6, "MotionMagic"=7, "MotionProfileArc"=10, "Disabled"=15] ("Control Mode")
        w465 = T13 0 items=["PercentOutput"=0, "Position"=1, "Velocity"=2, "Current"=3, "Follower"=5, "MotionProfile"=6, "MotionMagic"=7, "MotionProfileArc"=10, "Disabled"=15] ("Control Mode")
        n92 = call <vilib>:"WPI_SwitchGetLimitValue.vi"("error in (no error)"=w480, "SwitchDevRef"=w479) -> ("Switch Pressed"=w483:bool)  [unwired: 7 in, 2 out]
        n93 = call <vilib>:"WPI_SwitchGetLimitValue.vi"("error in (no error)"=w482, "SwitchDevRef"=w481) -> ("Switch Pressed"=w484:bool)  [unwired: 7 in, 2 out]
        n94 = Greater?(x=w485, y=20) -> (0:w486:bool)
        n95 = Not(x=w483) -> (.not. x?=w468:bool)
        "Intake 3" <- w468
        n96 = Not(x=w484) -> (.not. x?=w476:bool)
        "Elevate 3" <- w476
        n97 = Wait (ms)(milliseconds to wait=u32 100) -> ()  [unwired: 1 out]
        n98 = case shown="True" w476 {
          tunnel: [0.75 ("Output") w505] -> w475
          tunnel: w468 -> [_ w502]
          tunnel: [0.75 ("Output") w504] -> w467
          tunnel: [-0.1 ("Output") w503] -> w466
          tunnel: [FALSE ("Middle Thumb") w501] -> w462
          tunnel: [0.0 ("Z") w500] -> w461
          tunnel: [0.0 ("Y") w499] -> w460
          tunnel: [0.0 ("X") w498] -> w459
          tunnel: [WPI_SolenoidValue."Reverse" ("Value") w497] -> w458
          frame False {
          }
          frame True {
            n99 = case shown="False" w502 {
              tunnel: [0.75 ("Output") 0.0 ("Output")] -> w505
              tunnel: [0.75 ("Output") -0.75 ("Output")] -> w504
              tunnel: [0.0 ("Output") 0.0 ("Output")] -> w503
              tunnel: [FALSE ("Middle Thumb") FALSE ("Middle Thumb")] -> w501
              tunnel: [0.0 ("Z") 0.0 ("Z")] -> w500
              tunnel: [-0.3 ("Y") 0.0 ("Y")] -> w499
              tunnel: [0.0 ("X") 0.0 ("X")] -> w498
              tunnel: [WPI_SolenoidValue."Reverse" ("Value") WPI_SolenoidValue."Forward" ("Value")] -> w497
              frame False {
              }
              frame True {
              }
            }
          }
        }
        n100 = call-poly <vilib>:"WPI_SolenoidSet.vi"("error in (no error)"=w478, "Value"=w458, "SolenoidDevRef"=w477) -> ("error out"=w446:errorcluster, "SolenoidDevRef"=w447:T7)  [unwired: 7 in]
        n101 = call <vilib>:"CTRE_Phoenix_MotorControl_Set.vi"("error in (no error)"=w470, "Output"=w475, "Control Mode"=w463, "PhoenixMotorControlDevRef"=w469) -> ("error out"=w455:errorcluster, "PhoenixMotorControlDevRef"=w454:T9)  [unwired: 6 in]
        n102 = call <vilib>:"CTRE_Phoenix_MotorControl_Set.vi"("error in (no error)"=w472, "Output"=w467, "Control Mode"=w464, "PhoenixMotorControlDevRef"=w471) -> ()  [unwired: 6 in, 2 out]
        n103 = call <vilib>:"CTRE_Phoenix_MotorControl_Set.vi"("error in (no error)"=w474, "Output"=w466, "Control Mode"=w465, "PhoenixMotorControlDevRef"=w473) -> ("error out"=w457:errorcluster, "PhoenixMotorControlDevRef"=w456:T9)  [unwired: 6 in]
        n104 = call <vilib>:"CTRE_Phoenix_MotorControl_Set.vi"("error in (no error)"=w453, "Output"=-0.55, "Control Mode"=w451, "PhoenixMotorControlDevRef"=w452) -> ("error out"=w449:errorcluster, "PhoenixMotorControlDevRef"=w448:T9)  [unwired: 6 in]
        n105 = call "Drive_Vi.vi"("Middle Thumb"=w462, "Z"=w461, "Y"=w460, "X"=w459) -> ()  [unwired: 8 in]
      }
      n106 = call <vilib>:"WPI_SwitchRefNum Registry Get.vi"("refnum name"="Orange Limit Switch") -> ("error out"=w318:errorcluster, "SwitchDevRef"=w317:T4)  [unwired: 9 in]
      n107 = call <vilib>:"WPI_SwitchRefNum Registry Get.vi"("refnum name"="Blue Limit Switch") -> ("error out"=w320:errorcluster, "SwitchDevRef"=w319:T4)  [unwired: 9 in]
      n108 = while {
        tunnel: w310 -> [w445]
        tunnel: w309 -> [w444]
        tunnel: w320 -> [w441]
        tunnel: w319 -> [w440]
        tunnel: w318 -> [w439]
        tunnel: w317 -> [w438]
        tunnel: w316 -> [w413]
        tunnel: w315 -> [w412]
        tunnel: w314 -> [w403]
        tunnel: w313 -> [w404]
        tunnel: [w419] -> w308
        tunnel: [w418] -> w307
        tunnel: [w417] -> w306
        tunnel: [w416] -> w305
        tunnel: [w415] -> w304
        tunnel: [w414] -> w303
        tunnel: [w413] -> w302
        tunnel: [w412] -> w301
        tunnel: w300 -> [w411]
        tunnel: w299 -> [w410]
        tunnel: [w408] -> w298
        tunnel: [w407] -> w297
        tunnel: [w406] -> w296
        tunnel: [w405] -> w295
        i -> [w426]
        stop <- w424 stop-if-true
        w402 = T13 0 items=["PercentOutput"=0, "Position"=1, "Velocity"=2, "Current"=3, "Follower"=5, "MotionProfile"=6, "MotionMagic"=7, "MotionProfileArc"=10, "Disabled"=15] ("Control Mode")
        w425 = T13 0 items=["PercentOutput"=0, "Position"=1, "Velocity"=2, "Current"=3, "Follower"=5, "MotionProfile"=6, "MotionMagic"=7, "MotionProfileArc"=10, "Disabled"=15] ("Control Mode")
        n109 = call-poly <vilib>:"WPI_SolenoidSet.vi"("error in (no error)"=w410, "Value"=WPI_SolenoidValue."Forward", "SolenoidDevRef"=w411) -> ("error out"=w407:errorcluster, "SolenoidDevRef"=w408:T7)  [unwired: 7 in]
        n110 = call <vilib>:"WPI_SwitchGetLimitValue.vi"("error in (no error)"=w439, "SwitchDevRef"=w438) -> ("error out"=w416:errorcluster, "Switch Pressed"=w437:bool, "SwitchDevRef"=w417:T4)  [unwired: 7 in]
        "Orange Limit Pressed 5" <- w437
        n111 = call <vilib>:"WPI_SwitchGetLimitValue.vi"("error in (no error)"=w441, "SwitchDevRef"=w440) -> ("error out"=w418:errorcluster, "Switch Pressed"=w436:bool, "SwitchDevRef"=w419:T4)  [unwired: 7 in]
        "Blue Limit Pressed 5" <- w436
        n112 = call-poly <vilib>:"NT Read Value.vi"("Default Value"=0.0, "Name"="/limelight-drtrain/ty") -> ("Numeric"=w430:dbl)  [unwired: 8 in, 1 out]
        "Ty 5" <- w430
        n113 = Greater?(x=w426, y=5) -> (0:w424:bool)
        n114 = call "Turret_Aim.vi"("View Button"=FALSE ("Driver Right Thumb"), "Left Trigger"=2.0, "Orange Limit Pressed"=w436, "Blue Limit Pressed"=w437, "Right Bumper"=FALSE, "Left Bumper"=FALSE) -> ()  [unwired: 6 in]
        n115 = call "Shooter_Equation.vi"("Right Trigger"=2.0, "Ty"=w430) -> ("% voltage"=w433:dbl)  [unwired: 9 in]
        n116 = Wait (ms)(milliseconds to wait=u32 100) -> ()  [unwired: 1 out]
        n117 = call "Drive_Vi.vi"("Middle Thumb"=FALSE, "Z"=0.0, "Y"=0.15, "X"=0.0) -> ()  [unwired: 8 in]
        n118 = call <vilib>:"CTRE_Phoenix_MotorControl_Set.vi"("error in (no error)"=w403, "Output"=0.0, "Control Mode"=w402, "PhoenixMotorControlDevRef"=w404) -> ("error out"=w405:errorcluster, "PhoenixMotorControlDevRef"=w406:T9)  [unwired: 6 in]
        n119 = call <vilib>:"CTRE_Phoenix_MotorControl_Set.vi"("error in (no error)"=w445, "Output"=w433, "Control Mode"=w425, "PhoenixMotorControlDevRef"=w444) -> ("error out"=w415:errorcluster, "PhoenixMotorControlDevRef"=w414:T9)  [unwired: 6 in]
      }
      n120 = while {
        tunnel: w304 -> [w400]
        tunnel: w303 -> [w399]
        tunnel: w307 -> [w396]
        tunnel: w308 -> [w395]
        tunnel: w305 -> [w394]
        tunnel: w302 -> [w379]
        tunnel: w301 -> [w378]
        tunnel: w295 -> [w377]
        tunnel: w296 -> [w376]
        tunnel: w306 -> [w367]
        tunnel: w298 -> [w366]
        tunnel: w297 -> [w365]
        tunnel: [w363] -> w294
        tunnel: [w362] -> w293
        tunnel: [w361] -> w292
        tunnel: [w360] -> w291
        tunnel: [w359] -> w290
        tunnel: [w358] -> w289
        i -> [w382]
        stop <- w380 stop-if-true
        w374 = T13 0 items=["PercentOutput"=0, "Position"=1, "Velocity"=2, "Current"=3, "Follower"=5, "MotionProfile"=6, "MotionMagic"=7, "MotionProfileArc"=10, "Disabled"=15] ("Control Mode")
        w375 = T13 0 items=["PercentOutput"=0, "Position"=1, "Velocity"=2, "Current"=3, "Follower"=5, "MotionProfile"=6, "MotionMagic"=7, "MotionProfileArc"=10, "Disabled"=15] ("Control Mode")
        w381 = T13 0 items=["PercentOutput"=0, "Position"=1, "Velocity"=2, "Current"=3, "Follower"=5, "MotionProfile"=6, "MotionMagic"=7, "MotionProfileArc"=10, "Disabled"=15] ("Control Mode")
        n121 = call-poly <vilib>:"WPI_SolenoidSet.vi"("error in (no error)"=w365, "Value"=WPI_SolenoidValue."Off", "SolenoidDevRef"=w366) -> ()  [unwired: 7 in, 2 out]
        n122 = call <vilib>:"WPI_SwitchGetLimitValue.vi"("error in (no error)"=w394, "SwitchDevRef"=w367) -> ("Switch Pressed"=w393:bool)  [unwired: 7 in, 2 out]
        "Orange Limit Pressed 6" <- w393
        n123 = call <vilib>:"WPI_SwitchGetLimitValue.vi"("error in (no error)"=w396, "SwitchDevRef"=w395) -> ("Switch Pressed"=w392:bool)  [unwired: 7 in, 2 out]
        "Blue Limit Pressed 6" <- w392
        n124 = call-poly <vilib>:"NT Read Value.vi"("Default Value"=0.0, "Name"="/limelight-drtrain/ty") -> ("Numeric"=w386:dbl)  [unwired: 8 in, 1 out]
        "Ty 6" <- w386
        n125 = Greater?(x=w382, y=50) -> (0:w380:bool)
        n126 = call "Turret_Aim.vi"("View Button"=FALSE ("Driver Right Thumb"), "Left Trigger"=2.0, "Orange Limit Pressed"=w392, "Blue Limit Pressed"=w393, "Right Bumper"=FALSE, "Left Bumper"=FALSE) -> ()  [unwired: 6 in]
        n127 = call "Shooter_Equation.vi"("Right Trigger"=2.0, "Ty"=w386) -> ("% voltage"=w389:dbl)  [unwired: 9 in]
        n128 = Wait (ms)(milliseconds to wait=u32 100) -> ()  [unwired: 1 out]
        n129 = call "Drive_Vi.vi"("Middle Thumb"=FALSE, "Z"=0.0, "Y"=0.15, "X"=0.0) -> ()  [unwired: 8 in]
        n130 = call <vilib>:"CTRE_Phoenix_MotorControl_Set.vi"("error in (no error)"=w400, "Output"=w389, "Control Mode"=w381, "PhoenixMotorControlDevRef"=w399) -> ("error out"=w358:errorcluster, "PhoenixMotorControlDevRef"=w359:T9)  [unwired: 6 in]
        n131 = call <vilib>:"CTRE_Phoenix_MotorControl_Set.vi"("error in (no error)"=w377, "Output"=0.35, "Control Mode"=w374, "PhoenixMotorControlDevRef"=w376) -> ("error out"=w363:errorcluster, "PhoenixMotorControlDevRef"=w362:T9)  [unwired: 6 in]
        n132 = call <vilib>:"CTRE_Phoenix_MotorControl_Set.vi"("error in (no error)"=w379, "Output"=-0.35, "Control Mode"=w375, "PhoenixMotorControlDevRef"=w378) -> ("error out"=w360:errorcluster, "PhoenixMotorControlDevRef"=w361:T9)  [unwired: 6 in]
      }
      n133 = while {
        tunnel: w294 -> [w352]
        tunnel: w293 -> [w351]
        tunnel: w292 -> [w350]
        tunnel: w291 -> [w349]
        tunnel: w290 -> [w348]
        tunnel: w289 -> [w347]
        i -> [w344]
        stop <- w343 stop-if-true
        w355 = T13 0 items=["PercentOutput"=0, "Position"=1, "Velocity"=2, "Current"=3, "Follower"=5, "MotionProfile"=6, "MotionMagic"=7, "MotionProfileArc"=10, "Disabled"=15] ("Control Mode")
        w356 = T13 0 items=["PercentOutput"=0, "Position"=1, "Velocity"=2, "Current"=3, "Follower"=5, "MotionProfile"=6, "MotionMagic"=7, "MotionProfileArc"=10, "Disabled"=15] ("Control Mode")
        w357 = T13 0 items=["PercentOutput"=0, "Position"=1, "Velocity"=2, "Current"=3, "Follower"=5, "MotionProfile"=6, "MotionMagic"=7, "MotionProfileArc"=10, "Disabled"=15] ("Control Mode")
        n134 = call <vilib>:"CTRE_Phoenix_MotorControl_Set.vi"("error in (no error)"=w347, "Output"=0.0, "Control Mode"=w357, "PhoenixMotorControlDevRef"=w348) -> ()  [unwired: 6 in, 2 out]
        n135 = call <vilib>:"CTRE_Phoenix_MotorControl_Set.vi"("error in (no error)"=w352, "Output"=0.0, "Control Mode"=w355, "PhoenixMotorControlDevRef"=w351) -> ()  [unwired: 6 in, 2 out]
        n136 = call <vilib>:"CTRE_Phoenix_MotorControl_Set.vi"("error in (no error)"=w349, "Output"=0.0, "Control Mode"=w356, "PhoenixMotorControlDevRef"=w350) -> ()  [unwired: 6 in, 2 out]
        n137 = Greater?(x=w344, y=50) -> (0:w343:bool)
        n138 = Wait (ms)(milliseconds to wait=u32 100) -> ()  [unwired: 1 out]
      }
    }
    frame "2 Ball" {
      # "Pigeon Set"
      n139 = while {
        i -> [w768]
        stop <- w769 stop-if-true
        n140 = Wait (ms)(milliseconds to wait=u32 20) -> ()  [unwired: 1 out]
        n141 = Greater?(x=w768, y=2) -> (0:w769:bool)
        n142 = call "Drive_Vi.vi"("Middle Thumb"=TRUE, "Z"=0.0, "Y"=0.0, "X"=0.0) -> ()  [unwired: 8 in]
      }
      n143 = call <vilib>:"WPI_SwitchRefNum Registry Get.vi"("refnum name"="Intake Sensor") -> ("error out"=w573:errorcluster, "SwitchDevRef"=w572:T4)  [unwired: 9 in]
      n144 = call <vilib>:"WPI_SolenoidRefNum Registry Get.vi"("refnum name"="Intake Solenoid") -> ("error out"=w571:errorcluster, "SolenoidDevRef"=w570:T7)  [unwired: 9 in]
      n145 = call <vilib>:"CTRE_Phoenix_MotorControl_RefNumRegistryGet.vi"("refnum name"="Intake") -> ("error out"=w565:errorcluster, "PhoenixMotorControlDevRef"=w564:T9)  [unwired: 9 in]
      n146 = call <vilib>:"CTRE_Phoenix_MotorControl_RefNumRegistryGet.vi"("refnum name"="Reject") -> ("error out"=w567:errorcluster, "PhoenixMotorControlDevRef"=w566:T9)  [unwired: 9 in]
      n147 = call "Limit_Switches.vi"() -> ()  [unwired: 10 in, 2 out]
      n148 = call <vilib>:"CTRE_Phoenix_MotorControl_RefNumRegistryGet.vi"("refnum name"="Elevate") -> ("error out"=w569:errorcluster, "PhoenixMotorControlDevRef"=w568:T9)  [unwired: 9 in]
      n149 = call <vilib>:"WPI_SwitchRefNum Registry Get.vi"("refnum name"="Elevate Sensor") -> ("error out"=w575:errorcluster, "SwitchDevRef"=w574:T4)  [unwired: 9 in]
      n150 = call <vilib>:"CTRE_Phoenix_MotorControl_RefNumRegistryGet.vi"("refnum name"="Shoot") -> ("error out"=w553:errorcluster, "PhoenixMotorControlDevRef"=w552:T9)  [unwired: 9 in]
      n151 = while {
        tunnel: w575 -> [w723]
        tunnel: w574 -> [w722]
        tunnel: w573 -> [w721]
        tunnel: w572 -> [w720]
        tunnel: w571 -> [w719]
        tunnel: w570 -> [w718]
        tunnel: w569 -> [w715]
        tunnel: w568 -> [w714]
        tunnel: w567 -> [w713]
        tunnel: w566 -> [w712]
        tunnel: w565 -> [w711]
        tunnel: w564 -> [w710]
        tunnel: [w698] -> w557
        tunnel: [w697] -> w556
        tunnel: [w696] -> w555
        tunnel: [w695] -> w554
        tunnel: w553 -> [w694]
        tunnel: w552 -> [w693]
        tunnel: [w690] -> w551
        tunnel: [w689] -> w550
        tunnel: [w688] -> w541
        tunnel: [w687] -> w540
        i -> [w726]
        stop <- w727 stop-if-true
        w692 = T13 0 items=["PercentOutput"=0, "Position"=1, "Velocity"=2, "Current"=3, "Follower"=5, "MotionProfile"=6, "MotionMagic"=7, "MotionProfileArc"=10, "Disabled"=15] ("Control Mode")
        w704 = T13 0 items=["PercentOutput"=0, "Position"=1, "Velocity"=2, "Current"=3, "Follower"=5, "MotionProfile"=6, "MotionMagic"=7, "MotionProfileArc"=10, "Disabled"=15] ("Control Mode")
        w705 = T13 0 items=["PercentOutput"=0, "Position"=1, "Velocity"=2, "Current"=3, "Follower"=5, "MotionProfile"=6, "MotionMagic"=7, "MotionProfileArc"=10, "Disabled"=15] ("Control Mode")
        w706 = T13 0 items=["PercentOutput"=0, "Position"=1, "Velocity"=2, "Current"=3, "Follower"=5, "MotionProfile"=6, "MotionMagic"=7, "MotionProfileArc"=10, "Disabled"=15] ("Control Mode")
        n152 = call <vilib>:"WPI_SwitchGetLimitValue.vi"("error in (no error)"=w721, "SwitchDevRef"=w720) -> ("Switch Pressed"=w724:bool)  [unwired: 7 in, 2 out]
        n153 = call <vilib>:"WPI_SwitchGetLimitValue.vi"("error in (no error)"=w723, "SwitchDevRef"=w722) -> ("Switch Pressed"=w725:bool)  [unwired: 7 in, 2 out]
        n154 = Greater?(x=w726, y=20) -> (0:w727:bool)
        n155 = Not(x=w724) -> (.not. x?=w709:bool)
        "Intake" <- w709
        n156 = Not(x=w725) -> (.not. x?=w717:bool)
        "Elevate" <- w717
        n157 = Wait (ms)(milliseconds to wait=u32 100) -> ()  [unwired: 1 out]
        n158 = case shown="True" w717 {
          tunnel: [0.75 ("Output") w746] -> w716
          tunnel: w709 -> [_ w743]
          tunnel: [0.75 ("Output") w745] -> w708
          tunnel: [-0.1 ("Output") w744] -> w707
          tunnel: [FALSE ("Middle Thumb") w742] -> w703
          tunnel: [0.0 ("Z") w741] -> w702
          tunnel: [0.0 ("Y") w740] -> w701
          tunnel: [0.0 ("X") w739] -> w700
          tunnel: [WPI_SolenoidValue."Reverse" ("Value") w738] -> w699
          frame False {
          }
          frame True {
            n159 = case shown="False" w743 {
              tunnel: [0.75 ("Output") 0.0 ("Output")] -> w746
              tunnel: [0.0 ("Output") 0.0 ("Output")] -> w745
              tunnel: [0.0 ("Output") 0.0 ("Output")] -> w744
              tunnel: [FALSE ("Middle Thumb") FALSE ("Middle Thumb")] -> w742
              tunnel: [0.0 ("Z") 0.0 ("Z")] -> w741
              tunnel: [-0.3 ("Y") 0.0 ("Y")] -> w740
              tunnel: [0.0 ("X") 0.0 ("X")] -> w739
              tunnel: [WPI_SolenoidValue."Reverse" ("Value") WPI_SolenoidValue."Forward" ("Value")] -> w738
              frame False {
              }
              frame True {
              }
            }
          }
        }
        n160 = call-poly <vilib>:"WPI_SolenoidSet.vi"("error in (no error)"=w719, "Value"=w699, "SolenoidDevRef"=w718) -> ("error out"=w687:errorcluster, "SolenoidDevRef"=w688:T7)  [unwired: 7 in]
        n161 = call <vilib>:"CTRE_Phoenix_MotorControl_Set.vi"("error in (no error)"=w711, "Output"=w716, "Control Mode"=w704, "PhoenixMotorControlDevRef"=w710) -> ("error out"=w696:errorcluster, "PhoenixMotorControlDevRef"=w695:T9)  [unwired: 6 in]
        n162 = call <vilib>:"CTRE_Phoenix_MotorControl_Set.vi"("error in (no error)"=w713, "Output"=w708, "Control Mode"=w705, "PhoenixMotorControlDevRef"=w712) -> ()  [unwired: 6 in, 2 out]
        n163 = call <vilib>:"CTRE_Phoenix_MotorControl_Set.vi"("error in (no error)"=w715, "Output"=w707, "Control Mode"=w706, "PhoenixMotorControlDevRef"=w714) -> ("error out"=w698:errorcluster, "PhoenixMotorControlDevRef"=w697:T9)  [unwired: 6 in]
        n164 = call <vilib>:"CTRE_Phoenix_MotorControl_Set.vi"("error in (no error)"=w694, "Output"=-0.55, "Control Mode"=w692, "PhoenixMotorControlDevRef"=w693) -> ("error out"=w690:errorcluster, "PhoenixMotorControlDevRef"=w689:T9)  [unwired: 6 in]
        n165 = call "Drive_Vi.vi"("Middle Thumb"=w703, "Z"=w702, "Y"=w701, "X"=w700) -> ()  [unwired: 8 in]
      }
      n166 = call <vilib>:"WPI_SwitchRefNum Registry Get.vi"("refnum name"="Orange Limit Switch") -> ("error out"=w559:errorcluster, "SwitchDevRef"=w558:T4)  [unwired: 9 in]
      n167 = call <vilib>:"WPI_SwitchRefNum Registry Get.vi"("refnum name"="Blue Limit Switch") -> ("error out"=w561:errorcluster, "SwitchDevRef"=w560:T4)  [unwired: 9 in]
      n168 = while {
        tunnel: w551 -> [w686]
        tunnel: w550 -> [w685]
        tunnel: w561 -> [w682]
        tunnel: w560 -> [w681]
        tunnel: w559 -> [w680]
        tunnel: w558 -> [w679]
        tunnel: w557 -> [w654]
        tunnel: w556 -> [w653]
        tunnel: w555 -> [w644]
        tunnel: w554 -> [w645]
        tunnel: [w660] -> w549
        tunnel: [w659] -> w548
        tunnel: [w658] -> w547
        tunnel: [w657] -> w546
        tunnel: [w656] -> w545
        tunnel: [w655] -> w544
        tunnel: [w654] -> w543
        tunnel: [w653] -> w542
        tunnel: w541 -> [w652]
        tunnel: w540 -> [w651]
        tunnel: [w649] -> w539
        tunnel: [w648] -> w538
        tunnel: [w647] -> w537
        tunnel: [w646] -> w536
        i -> [w667]
        stop <- w665 stop-if-true
        w643 = T13 0 items=["PercentOutput"=0, "Position"=1, "Velocity"=2, "Current"=3, "Follower"=5, "MotionProfile"=6, "MotionMagic"=7, "MotionProfileArc"=10, "Disabled"=15] ("Control Mode")
        w666 = T13 0 items=["PercentOutput"=0, "Position"=1, "Velocity"=2, "Current"=3, "Follower"=5, "MotionProfile"=6, "MotionMagic"=7, "MotionProfileArc"=10, "Disabled"=15] ("Control Mode")
        n169 = call-poly <vilib>:"WPI_SolenoidSet.vi"("error in (no error)"=w651, "Value"=WPI_SolenoidValue."Forward", "SolenoidDevRef"=w652) -> ("error out"=w648:errorcluster, "SolenoidDevRef"=w649:T7)  [unwired: 7 in]
        n170 = call <vilib>:"WPI_SwitchGetLimitValue.vi"("error in (no error)"=w680, "SwitchDevRef"=w679) -> ("error out"=w657:errorcluster, "Switch Pressed"=w678:bool, "SwitchDevRef"=w658:T4)  [unwired: 7 in]
        "Orange Limit Pressed" <- w678
        n171 = call <vilib>:"WPI_SwitchGetLimitValue.vi"("error in (no error)"=w682, "SwitchDevRef"=w681) -> ("error out"=w659:errorcluster, "Switch Pressed"=w677:bool, "SwitchDevRef"=w660:T4)  [unwired: 7 in]
        "Blue Limit Pressed" <- w677
        n172 = call-poly <vilib>:"NT Read Value.vi"("Default Value"=0.0, "Name"="/limelight-drtrain/ty") -> ("Numeric"=w671:dbl)  [unwired: 8 in, 1 out]
        "Ty" <- w671
        n173 = Greater?(x=w667, y=5) -> (0:w665:bool)
        n174 = call "Turret_Aim.vi"("View Button"=FALSE ("Driver Right Thumb"), "Left Trigger"=2.0, "Orange Limit Pressed"=w677, "Blue Limit Pressed"=w678, "Right Bumper"=FALSE, "Left Bumper"=FALSE) -> ()  [unwired: 6 in]
        n175 = call "Shooter_Equation.vi"("Right Trigger"=2.0, "Ty"=w671) -> ("% voltage"=w674:dbl)  [unwired: 9 in]
        n176 = Wait (ms)(milliseconds to wait=u32 100) -> ()  [unwired: 1 out]
        n177 = call "Drive_Vi.vi"("Middle Thumb"=FALSE, "Z"=0.0, "Y"=0.15, "X"=0.0) -> ()  [unwired: 8 in]
        n178 = call <vilib>:"CTRE_Phoenix_MotorControl_Set.vi"("error in (no error)"=w644, "Output"=0.0, "Control Mode"=w643, "PhoenixMotorControlDevRef"=w645) -> ("error out"=w646:errorcluster, "PhoenixMotorControlDevRef"=w647:T9)  [unwired: 6 in]
        n179 = call <vilib>:"CTRE_Phoenix_MotorControl_Set.vi"("error in (no error)"=w686, "Output"=w674, "Control Mode"=w666, "PhoenixMotorControlDevRef"=w685) -> ("error out"=w656:errorcluster, "PhoenixMotorControlDevRef"=w655:T9)  [unwired: 6 in]
      }
      n180 = while {
        tunnel: w545 -> [w641]
        tunnel: w544 -> [w640]
        tunnel: w548 -> [w637]
        tunnel: w549 -> [w636]
        tunnel: w546 -> [w635]
        tunnel: w543 -> [w620]
        tunnel: w542 -> [w619]
        tunnel: w536 -> [w618]
        tunnel: w537 -> [w617]
        tunnel: w547 -> [w608]
        tunnel: w539 -> [w607]
        tunnel: w538 -> [w606]
        tunnel: [w604] -> w535
        tunnel: [w603] -> w534
        tunnel: [w602] -> w533
        tunnel: [w601] -> w532
        tunnel: [w600] -> w531
        tunnel: [w599] -> w530
        i -> [w623]
        stop <- w621 stop-if-true
        w615 = T13 0 items=["PercentOutput"=0, "Position"=1, "Velocity"=2, "Current"=3, "Follower"=5, "MotionProfile"=6, "MotionMagic"=7, "MotionProfileArc"=10, "Disabled"=15] ("Control Mode")
        w616 = T13 0 items=["PercentOutput"=0, "Position"=1, "Velocity"=2, "Current"=3, "Follower"=5, "MotionProfile"=6, "MotionMagic"=7, "MotionProfileArc"=10, "Disabled"=15] ("Control Mode")
        w622 = T13 0 items=["PercentOutput"=0, "Position"=1, "Velocity"=2, "Current"=3, "Follower"=5, "MotionProfile"=6, "MotionMagic"=7, "MotionProfileArc"=10, "Disabled"=15] ("Control Mode")
        n181 = call-poly <vilib>:"WPI_SolenoidSet.vi"("error in (no error)"=w606, "Value"=WPI_SolenoidValue."Off", "SolenoidDevRef"=w607) -> ()  [unwired: 7 in, 2 out]
        n182 = call <vilib>:"WPI_SwitchGetLimitValue.vi"("error in (no error)"=w635, "SwitchDevRef"=w608) -> ("Switch Pressed"=w634:bool)  [unwired: 7 in, 2 out]
        "Orange Limit Pressed 2" <- w634
        n183 = call <vilib>:"WPI_SwitchGetLimitValue.vi"("error in (no error)"=w637, "SwitchDevRef"=w636) -> ("Switch Pressed"=w633:bool)  [unwired: 7 in, 2 out]
        "Blue Limit Pressed 2" <- w633
        n184 = call-poly <vilib>:"NT Read Value.vi"("Default Value"=0.0, "Name"="/limelight-drtrain/ty") -> ("Numeric"=w627:dbl)  [unwired: 8 in, 1 out]
        "Ty 2" <- w627
        n185 = Greater?(x=w623, y=50) -> (0:w621:bool)
        n186 = call "Turret_Aim.vi"("View Button"=FALSE ("Driver Right Thumb"), "Left Trigger"=2.0, "Orange Limit Pressed"=w633, "Blue Limit Pressed"=w634, "Right Bumper"=FALSE, "Left Bumper"=FALSE) -> ()  [unwired: 6 in]
        n187 = call "Shooter_Equation.vi"("Right Trigger"=2.0, "Ty"=w627) -> ("% voltage"=w630:dbl)  [unwired: 9 in]
        n188 = Wait (ms)(milliseconds to wait=u32 100) -> ()  [unwired: 1 out]
        n189 = call "Drive_Vi.vi"("Middle Thumb"=FALSE, "Z"=0.0, "Y"=0.15, "X"=0.0) -> ()  [unwired: 8 in]
        n190 = call <vilib>:"CTRE_Phoenix_MotorControl_Set.vi"("error in (no error)"=w641, "Output"=w630, "Control Mode"=w622, "PhoenixMotorControlDevRef"=w640) -> ("error out"=w599:errorcluster, "PhoenixMotorControlDevRef"=w600:T9)  [unwired: 6 in]
        n191 = call <vilib>:"CTRE_Phoenix_MotorControl_Set.vi"("error in (no error)"=w618, "Output"=0.35, "Control Mode"=w615, "PhoenixMotorControlDevRef"=w617) -> ("error out"=w604:errorcluster, "PhoenixMotorControlDevRef"=w603:T9)  [unwired: 6 in]
        n192 = call <vilib>:"CTRE_Phoenix_MotorControl_Set.vi"("error in (no error)"=w620, "Output"=-0.35, "Control Mode"=w616, "PhoenixMotorControlDevRef"=w619) -> ("error out"=w601:errorcluster, "PhoenixMotorControlDevRef"=w602:T9)  [unwired: 6 in]
      }
      n193 = while {
        tunnel: w535 -> [w593]
        tunnel: w534 -> [w592]
        tunnel: w533 -> [w591]
        tunnel: w532 -> [w590]
        tunnel: w531 -> [w589]
        tunnel: w530 -> [w588]
        i -> [w585]
        stop <- w584 stop-if-true
        w596 = T13 0 items=["PercentOutput"=0, "Position"=1, "Velocity"=2, "Current"=3, "Follower"=5, "MotionProfile"=6, "MotionMagic"=7, "MotionProfileArc"=10, "Disabled"=15] ("Control Mode")
        w597 = T13 0 items=["PercentOutput"=0, "Position"=1, "Velocity"=2, "Current"=3, "Follower"=5, "MotionProfile"=6, "MotionMagic"=7, "MotionProfileArc"=10, "Disabled"=15] ("Control Mode")
        w598 = T13 0 items=["PercentOutput"=0, "Position"=1, "Velocity"=2, "Current"=3, "Follower"=5, "MotionProfile"=6, "MotionMagic"=7, "MotionProfileArc"=10, "Disabled"=15] ("Control Mode")
        n194 = call <vilib>:"CTRE_Phoenix_MotorControl_Set.vi"("error in (no error)"=w588, "Output"=0.0, "Control Mode"=w598, "PhoenixMotorControlDevRef"=w589) -> ()  [unwired: 6 in, 2 out]
        n195 = call <vilib>:"CTRE_Phoenix_MotorControl_Set.vi"("error in (no error)"=w593, "Output"=0.0, "Control Mode"=w596, "PhoenixMotorControlDevRef"=w592) -> ()  [unwired: 6 in, 2 out]
        n196 = call <vilib>:"CTRE_Phoenix_MotorControl_Set.vi"("error in (no error)"=w590, "Output"=0.0, "Control Mode"=w597, "PhoenixMotorControlDevRef"=w591) -> ()  [unwired: 6 in, 2 out]
        n197 = Greater?(x=w585, y=50) -> (0:w584:bool)
        n198 = Wait (ms)(milliseconds to wait=u32 100) -> ()  [unwired: 1 out]
      }
    }
    frame "4 Ball Pos 1" {
      # "Get limelight position and shooter started up"
      # "Driving backwards, put arms down and running intake to get ball"
      n199 = for {
        N: 20 -> [_]
        n200 = global write "GlobalDriveJoysticks.vi" "Y"(-0.5 ("Y")) -> ()
        n201 = global write "GlobalDriveJoysticks.vi" "Middle Button"(FALSE ("Middle Thumb")) -> ()
        n202 = global write "GlobalDriveJoysticks.vi" "Z"(0.0 ("Z")) -> ()
        n203 = global write "GlobalDriveJoysticks.vi" "X"(0.0 ("X")) -> ()
        n204 = Wait (ms)(milliseconds to wait=u32 100) -> ()  [unwired: 1 out]
      }
    }
    frame "4 Ball Pos 2" {
      # "Pigeon Set"
      n205 = while {
        i -> [w1015]
        stop <- w1016 stop-if-true
        n206 = Wait (ms)(milliseconds to wait=u32 20) -> ()  [unwired: 1 out]
        n207 = Greater?(x=w1015, y=2) -> (0:w1016:bool)
        n208 = call "Drive_Vi.vi"("Middle Thumb"=TRUE, "Z"=0.0, "Y"=0.0, "X"=0.0) -> ()  [unwired: 8 in]
      }
      n209 = call <vilib>:"CTRE_Phoenix_MotorControl_RefNumRegistryGet.vi"("refnum name"="Elevate") -> ("error out"=w816:errorcluster, "PhoenixMotorControlDevRef"=w815:T9)  [unwired: 9 in]
      n210 = call <vilib>:"WPI_SwitchRefNum Registry Get.vi"("refnum name"="Intake Sensor") -> ("error out"=w820:errorcluster, "SwitchDevRef"=w819:T4)  [unwired: 9 in]
      n211 = call <vilib>:"CTRE_Phoenix_MotorControl_RefNumRegistryGet.vi"("refnum name"="Reject") -> ("error out"=w814:errorcluster, "PhoenixMotorControlDevRef"=w813:T9)  [unwired: 9 in]
      n212 = call <vilib>:"WPI_SwitchRefNum Registry Get.vi"("refnum name"="Elevate Sensor") -> ("error out"=w822:errorcluster, "SwitchDevRef"=w821:T4)  [unwired: 9 in]
      n213 = call <vilib>:"CTRE_Phoenix_MotorControl_RefNumRegistryGet.vi"("refnum name"="Shoot") -> ("error out"=w800:errorcluster, "PhoenixMotorControlDevRef"=w799:T9)  [unwired: 9 in]
      n214 = call <vilib>:"WPI_SolenoidRefNum Registry Get.vi"("refnum name"="Intake Solenoid") -> ("error out"=w818:errorcluster, "SolenoidDevRef"=w817:T7)  [unwired: 9 in]
      n215 = call <vilib>:"CTRE_Phoenix_MotorControl_RefNumRegistryGet.vi"("refnum name"="Intake") -> ("error out"=w812:errorcluster, "PhoenixMotorControlDevRef"=w811:T9)  [unwired: 9 in]
      n216 = call "Limit_Switches.vi"() -> ()  [unwired: 10 in, 2 out]
      n217 = while {
        tunnel: w822 -> [w970]
        tunnel: w821 -> [w969]
        tunnel: w820 -> [w968]
        tunnel: w819 -> [w967]
        tunnel: w818 -> [w966]
        tunnel: w817 -> [w965]
        tunnel: w816 -> [w962]
        tunnel: w815 -> [w961]
        tunnel: w814 -> [w960]
        tunnel: w813 -> [w959]
        tunnel: w812 -> [w958]
        tunnel: w811 -> [w957]
        tunnel: [w945] -> w804
        tunnel: [w944] -> w803
        tunnel: [w943] -> w802
        tunnel: [w942] -> w801
        tunnel: w800 -> [w941]
        tunnel: w799 -> [w940]
        tunnel: [w937] -> w798
        tunnel: [w936] -> w797
        tunnel: [w935] -> w788
        tunnel: [w934] -> w787
        i -> [w973]
        stop <- w974 stop-if-true
        w939 = T13 0 items=["PercentOutput"=0, "Position"=1, "Velocity"=2, "Current"=3, "Follower"=5, "MotionProfile"=6, "MotionMagic"=7, "MotionProfileArc"=10, "Disabled"=15] ("Control Mode")
        w951 = T13 0 items=["PercentOutput"=0, "Position"=1, "Velocity"=2, "Current"=3, "Follower"=5, "MotionProfile"=6, "MotionMagic"=7, "MotionProfileArc"=10, "Disabled"=15] ("Control Mode")
        w952 = T13 0 items=["PercentOutput"=0, "Position"=1, "Velocity"=2, "Current"=3, "Follower"=5, "MotionProfile"=6, "MotionMagic"=7, "MotionProfileArc"=10, "Disabled"=15] ("Control Mode")
        w953 = T13 0 items=["PercentOutput"=0, "Position"=1, "Velocity"=2, "Current"=3, "Follower"=5, "MotionProfile"=6, "MotionMagic"=7, "MotionProfileArc"=10, "Disabled"=15] ("Control Mode")
        n218 = call <vilib>:"WPI_SwitchGetLimitValue.vi"("error in (no error)"=w968, "SwitchDevRef"=w967) -> ("Switch Pressed"=w971:bool)  [unwired: 7 in, 2 out]
        n219 = call <vilib>:"WPI_SwitchGetLimitValue.vi"("error in (no error)"=w970, "SwitchDevRef"=w969) -> ("Switch Pressed"=w972:bool)  [unwired: 7 in, 2 out]
        n220 = Greater?(x=w973, y=20) -> (0:w974:bool)
        n221 = Not(x=w971) -> (.not. x?=w956:bool)
        "Intake 2" <- w956
        n222 = Not(x=w972) -> (.not. x?=w964:bool)
        "Elevate 2" <- w964
        n223 = Wait (ms)(milliseconds to wait=u32 100) -> ()  [unwired: 1 out]
        n224 = case shown="True" w964 {
          tunnel: [0.75 ("Output") w993] -> w963
          tunnel: w956 -> [_ w990]
          tunnel: [0.75 ("Output") w992] -> w955
          tunnel: [-0.1 ("Output") w991] -> w954
          tunnel: [FALSE ("Middle Thumb") w989] -> w950
          tunnel: [0.0 ("Z") w988] -> w949
          tunnel: [0.0 ("Y") w987] -> w948
          tunnel: [0.0 ("X") w986] -> w947
          tunnel: [WPI_SolenoidValue."Reverse" ("Value") w985] -> w946
          frame False {
          }
          frame True {
            n225 = case shown="True" w990 {
              tunnel: [0.75 ("Output") 0.0 ("Output")] -> w993
              tunnel: [0.0 ("Output") 0.0 ("Output")] -> w992
              tunnel: [0.0 ("Output") 0.0 ("Output")] -> w991
              tunnel: [FALSE ("Middle Thumb") FALSE ("Middle Thumb")] -> w989
              tunnel: [0.0 ("Z") 0.0 ("Z")] -> w988
              tunnel: [-0.3 ("Y") 0.0 ("Y")] -> w987
              tunnel: [0.0 ("X") 0.0 ("X")] -> w986
              tunnel: [WPI_SolenoidValue."Reverse" ("Value") WPI_SolenoidValue."Forward" ("Value")] -> w985
              frame False {
              }
              frame True {
              }
            }
          }
        }
        n226 = call-poly <vilib>:"WPI_SolenoidSet.vi"("error in (no error)"=w966, "Value"=w946, "SolenoidDevRef"=w965) -> ("error out"=w934:errorcluster, "SolenoidDevRef"=w935:T7)  [unwired: 7 in]
        n227 = call <vilib>:"CTRE_Phoenix_MotorControl_Set.vi"("error in (no error)"=w958, "Output"=w963, "Control Mode"=w951, "PhoenixMotorControlDevRef"=w957) -> ("error out"=w943:errorcluster, "PhoenixMotorControlDevRef"=w942:T9)  [unwired: 6 in]
        n228 = call <vilib>:"CTRE_Phoenix_MotorControl_Set.vi"("error in (no error)"=w960, "Output"=w955, "Control Mode"=w952, "PhoenixMotorControlDevRef"=w959) -> ()  [unwired: 6 in, 2 out]
        n229 = call <vilib>:"CTRE_Phoenix_MotorControl_Set.vi"("error in (no error)"=w962, "Output"=w954, "Control Mode"=w953, "PhoenixMotorControlDevRef"=w961) -> ("error out"=w945:errorcluster, "PhoenixMotorControlDevRef"=w944:T9)  [unwired: 6 in]
        n230 = call <vilib>:"CTRE_Phoenix_MotorControl_Set.vi"("error in (no error)"=w941, "Output"=-0.55, "Control Mode"=w939, "PhoenixMotorControlDevRef"=w940) -> ("error out"=w937:errorcluster, "PhoenixMotorControlDevRef"=w936:T9)  [unwired: 6 in]
        n231 = call "Drive_Vi.vi"("Middle Thumb"=w950, "Z"=w949, "Y"=w948, "X"=w947) -> ()  [unwired: 8 in]
      }
      n232 = call <vilib>:"WPI_SwitchRefNum Registry Get.vi"("refnum name"="Orange Limit Switch") -> ("error out"=w806:errorcluster, "SwitchDevRef"=w805:T4)  [unwired: 9 in]
      n233 = call <vilib>:"WPI_SwitchRefNum Registry Get.vi"("refnum name"="Blue Limit Switch") -> ("error out"=w808:errorcluster, "SwitchDevRef"=w807:T4)  [unwired: 9 in]
      n234 = while {
        tunnel: w798 -> [w933]
        tunnel: w797 -> [w932]
        tunnel: w808 -> [w929]
        tunnel: w807 -> [w928]
        tunnel: w806 -> [w927]
        tunnel: w805 -> [w926]
        tunnel: w804 -> [w901]
        tunnel: w803 -> [w900]
        tunnel: w802 -> [w891]
        tunnel: w801 -> [w892]
        tunnel: [w907] -> w796
        tunnel: [w906] -> w795
        tunnel: [w905] -> w794
        tunnel: [w904] -> w793
        tunnel: [w903] -> w792
        tunnel: [w902] -> w791
        tunnel: [w901] -> w790
        tunnel: [w900] -> w789
        tunnel: w788 -> [w899]
        tunnel: w787 -> [w898]
        tunnel: [w896] -> w786
        tunnel: [w895] -> w785
        tunnel: [w894] -> w784
        tunnel: [w893] -> w783
        i -> [w914]
        stop <- w912 stop-if-true
        w890 = T13 0 items=["PercentOutput"=0, "Position"=1, "Velocity"=2, "Current"=3, "Follower"=5, "MotionProfile"=6, "MotionMagic"=7, "MotionProfileArc"=10, "Disabled"=15] ("Control Mode")
        w913 = T13 0 items=["PercentOutput"=0, "Position"=1, "Velocity"=2, "Current"=3, "Follower"=5, "MotionProfile"=6, "MotionMagic"=7, "MotionProfileArc"=10, "Disabled"=15] ("Control Mode")
        n235 = call-poly <vilib>:"WPI_SolenoidSet.vi"("error in (no error)"=w898, "Value"=WPI_SolenoidValue."Forward", "SolenoidDevRef"=w899) -> ("error out"=w895:errorcluster, "SolenoidDevRef"=w896:T7)  [unwired: 7 in]
        n236 = call <vilib>:"WPI_SwitchGetLimitValue.vi"("error in (no error)"=w927, "SwitchDevRef"=w926) -> ("error out"=w904:errorcluster, "Switch Pressed"=w925:bool, "SwitchDevRef"=w905:T4)  [unwired: 7 in]
        "Orange Limit Pressed 3" <- w925
        n237 = call <vilib>:"WPI_SwitchGetLimitValue.vi"("error in (no error)"=w929, "SwitchDevRef"=w928) -> ("error out"=w906:errorcluster, "Switch Pressed"=w924:bool, "SwitchDevRef"=w907:T4)  [unwired: 7 in]
        "Blue Limit Pressed 3" <- w924
        n238 = call-poly <vilib>:"NT Read Value.vi"("Default Value"=0.0, "Name"="/limelight-drtrain/ty") -> ("Numeric"=w918:dbl)  [unwired: 8 in, 1 out]
        "Ty 3" <- w918
        n239 = Greater?(x=w914, y=5) -> (0:w912:bool)
        n240 = call "Turret_Aim.vi"("View Button"=FALSE ("Driver Right Thumb"), "Left Trigger"=2.0, "Orange Limit Pressed"=w924, "Blue Limit Pressed"=w925, "Right Bumper"=FALSE, "Left Bumper"=FALSE) -> ()  [unwired: 6 in]
        n241 = call "Shooter_Equation.vi"("Right Trigger"=2.0, "Ty"=w918) -> ("% voltage"=w921:dbl)  [unwired: 9 in]
        n242 = Wait (ms)(milliseconds to wait=u32 100) -> ()  [unwired: 1 out]
        n243 = call "Drive_Vi.vi"("Middle Thumb"=FALSE, "Z"=0.0, "Y"=0.15, "X"=0.0) -> ()  [unwired: 8 in]
        n244 = call <vilib>:"CTRE_Phoenix_MotorControl_Set.vi"("error in (no error)"=w891, "Output"=0.0, "Control Mode"=w890, "PhoenixMotorControlDevRef"=w892) -> ("error out"=w893:errorcluster, "PhoenixMotorControlDevRef"=w894:T9)  [unwired: 6 in]
        n245 = call <vilib>:"CTRE_Phoenix_MotorControl_Set.vi"("error in (no error)"=w933, "Output"=w921, "Control Mode"=w913, "PhoenixMotorControlDevRef"=w932) -> ("error out"=w903:errorcluster, "PhoenixMotorControlDevRef"=w902:T9)  [unwired: 6 in]
      }
      n246 = while {
        tunnel: w792 -> [w888]
        tunnel: w791 -> [w887]
        tunnel: w795 -> [w884]
        tunnel: w796 -> [w883]
        tunnel: w793 -> [w882]
        tunnel: w790 -> [w867]
        tunnel: w789 -> [w866]
        tunnel: w783 -> [w865]
        tunnel: w784 -> [w864]
        tunnel: w794 -> [w855]
        tunnel: w786 -> [w854]
        tunnel: w785 -> [w853]
        tunnel: [w851] -> w782
        tunnel: [w850] -> w781
        tunnel: [w849] -> w780
        tunnel: [w848] -> w779
        tunnel: [w847] -> w778
        tunnel: [w846] -> w777
        i -> [w870]
        stop <- w868 stop-if-true
        w862 = T13 0 items=["PercentOutput"=0, "Position"=1, "Velocity"=2, "Current"=3, "Follower"=5, "MotionProfile"=6, "MotionMagic"=7, "MotionProfileArc"=10, "Disabled"=15] ("Control Mode")
        w863 = T13 0 items=["PercentOutput"=0, "Position"=1, "Velocity"=2, "Current"=3, "Follower"=5, "MotionProfile"=6, "MotionMagic"=7, "MotionProfileArc"=10, "Disabled"=15] ("Control Mode")
        w869 = T13 0 items=["PercentOutput"=0, "Position"=1, "Velocity"=2, "Current"=3, "Follower"=5, "MotionProfile"=6, "MotionMagic"=7, "MotionProfileArc"=10, "Disabled"=15] ("Control Mode")
        n247 = call-poly <vilib>:"WPI_SolenoidSet.vi"("error in (no error)"=w853, "Value"=WPI_SolenoidValue."Off", "SolenoidDevRef"=w854) -> ()  [unwired: 7 in, 2 out]
        n248 = call <vilib>:"WPI_SwitchGetLimitValue.vi"("error in (no error)"=w882, "SwitchDevRef"=w855) -> ("Switch Pressed"=w881:bool)  [unwired: 7 in, 2 out]
        "Orange Limit Pressed 4" <- w881
        n249 = call <vilib>:"WPI_SwitchGetLimitValue.vi"("error in (no error)"=w884, "SwitchDevRef"=w883) -> ("Switch Pressed"=w880:bool)  [unwired: 7 in, 2 out]
        "Blue Limit Pressed 4" <- w880
        n250 = call-poly <vilib>:"NT Read Value.vi"("Default Value"=0.0, "Name"="/limelight-drtrain/ty") -> ("Numeric"=w874:dbl)  [unwired: 8 in, 1 out]
        "Ty 4" <- w874
        n251 = Greater?(x=w870, y=50) -> (0:w868:bool)
        n252 = call "Turret_Aim.vi"("View Button"=FALSE ("Driver Right Thumb"), "Left Trigger"=2.0, "Orange Limit Pressed"=w880, "Blue Limit Pressed"=w881, "Right Bumper"=FALSE, "Left Bumper"=FALSE) -> ()  [unwired: 6 in]
        n253 = call "Shooter_Equation.vi"("Right Trigger"=2.0, "Ty"=w874) -> ("% voltage"=w877:dbl)  [unwired: 9 in]
        n254 = Wait (ms)(milliseconds to wait=u32 100) -> ()  [unwired: 1 out]
        n255 = call "Drive_Vi.vi"("Middle Thumb"=FALSE, "Z"=0.0, "Y"=0.15, "X"=0.0) -> ()  [unwired: 8 in]
        n256 = call <vilib>:"CTRE_Phoenix_MotorControl_Set.vi"("error in (no error)"=w888, "Output"=w877, "Control Mode"=w869, "PhoenixMotorControlDevRef"=w887) -> ("error out"=w846:errorcluster, "PhoenixMotorControlDevRef"=w847:T9)  [unwired: 6 in]
        n257 = call <vilib>:"CTRE_Phoenix_MotorControl_Set.vi"("error in (no error)"=w865, "Output"=0.35, "Control Mode"=w862, "PhoenixMotorControlDevRef"=w864) -> ("error out"=w851:errorcluster, "PhoenixMotorControlDevRef"=w850:T9)  [unwired: 6 in]
        n258 = call <vilib>:"CTRE_Phoenix_MotorControl_Set.vi"("error in (no error)"=w867, "Output"=-0.35, "Control Mode"=w863, "PhoenixMotorControlDevRef"=w866) -> ("error out"=w848:errorcluster, "PhoenixMotorControlDevRef"=w849:T9)  [unwired: 6 in]
      }
      n259 = while {
        tunnel: w782 -> [w840]
        tunnel: w781 -> [w839]
        tunnel: w780 -> [w838]
        tunnel: w779 -> [w837]
        tunnel: w778 -> [w836]
        tunnel: w777 -> [w835]
        i -> [w832]
        stop <- w831 stop-if-true
        w843 = T13 0 items=["PercentOutput"=0, "Position"=1, "Velocity"=2, "Current"=3, "Follower"=5, "MotionProfile"=6, "MotionMagic"=7, "MotionProfileArc"=10, "Disabled"=15] ("Control Mode")
        w844 = T13 0 items=["PercentOutput"=0, "Position"=1, "Velocity"=2, "Current"=3, "Follower"=5, "MotionProfile"=6, "MotionMagic"=7, "MotionProfileArc"=10, "Disabled"=15] ("Control Mode")
        w845 = T13 0 items=["PercentOutput"=0, "Position"=1, "Velocity"=2, "Current"=3, "Follower"=5, "MotionProfile"=6, "MotionMagic"=7, "MotionProfileArc"=10, "Disabled"=15] ("Control Mode")
        n260 = call <vilib>:"CTRE_Phoenix_MotorControl_Set.vi"("error in (no error)"=w835, "Output"=0.0, "Control Mode"=w845, "PhoenixMotorControlDevRef"=w836) -> ()  [unwired: 6 in, 2 out]
        n261 = call <vilib>:"CTRE_Phoenix_MotorControl_Set.vi"("error in (no error)"=w840, "Output"=0.0, "Control Mode"=w843, "PhoenixMotorControlDevRef"=w839) -> ()  [unwired: 6 in, 2 out]
        n262 = call <vilib>:"CTRE_Phoenix_MotorControl_Set.vi"("error in (no error)"=w837, "Output"=0.0, "Control Mode"=w844, "PhoenixMotorControlDevRef"=w838) -> ()  [unwired: 6 in, 2 out]
        n263 = Greater?(x=w832, y=50) -> (0:w831:bool)
        n264 = Wait (ms)(milliseconds to wait=u32 100) -> ()  [unwired: 1 out]
      }
    }
    frame "4 Ball Pos 3" {
    }
    frame "Auton test" {
      w1027 = T13 0 items=["PercentOutput"=0, "Position"=1, "Velocity"=2, "Current"=3, "Follower"=5, "MotionProfile"=6, "MotionMagic"=7, "MotionProfileArc"=10, "Disabled"=15] ("Control Mode")
      w1041 = T13 0 items=["PercentOutput"=0, "Position"=1, "Velocity"=2, "Current"=3, "Follower"=5, "MotionProfile"=6, "MotionMagic"=7, "MotionProfileArc"=10, "Disabled"=15] ("Control Mode")
      w1019 = T13 0 items=["PercentOutput"=0, "Position"=1, "Velocity"=2, "Current"=3, "Follower"=5, "MotionProfile"=6, "MotionMagic"=7, "MotionProfileArc"=10, "Disabled"=15] ("Control Mode")
      w1044 = T13 0 items=["PercentOutput"=0, "Position"=1, "Velocity"=2, "Current"=3, "Follower"=5, "MotionProfile"=6, "MotionMagic"=7, "MotionProfileArc"=10, "Disabled"=15] ("Control Mode")
      n265 = call <vilib>:"CTRE_Phoenix_MotorControl_RefNumRegistryGet.vi"("refnum name"="Reject") -> ("error out"=w1043:errorcluster, "PhoenixMotorControlDevRef"=w1042:T9)  [unwired: 9 in]
      n266 = call <vilib>:"CTRE_Phoenix_MotorControl_RefNumRegistryGet.vi"("refnum name"="Intake") -> ("error out"=w1046:errorcluster, "PhoenixMotorControlDevRef"=w1045:T9)  [unwired: 9 in]
      n267 = call <vilib>:"CTRE_Phoenix_MotorControl_RefNumRegistryGet.vi"("refnum name"="Elevate") -> ("error out"=w1020:errorcluster, "PhoenixMotorControlDevRef"=w1018:T9)  [unwired: 9 in]
      n268 = call <vilib>:"CTRE_Phoenix_MotorControl_RefNumRegistryGet.vi"("refnum name"="Shoot") -> ("error out"=w1029:errorcluster, "PhoenixMotorControlDevRef"=w1026:T9)  [unwired: 9 in]
      n269 = call <vilib>:"WPI_SwitchRefNum Registry Get.vi"("refnum name"="Elevate Elevate") -> ("error out"=w1033:errorcluster, "SwitchDevRef"=w1032:T4)  [unwired: 9 in]
      n270 = call <vilib>:"WPI_SwitchRefNum Registry Get.vi"("refnum name"="Intake Sensor") -> ("error out"=w1031:errorcluster, "SwitchDevRef"=w1030:T4)  [unwired: 9 in]
      n271 = call <vilib>:"WPI_SwitchGetLimitValue.vi"("error in (no error)"=w1031, "SwitchDevRef"=w1030) -> ("Switch Pressed"=w1025:bool)  [unwired: 7 in, 2 out]
      n272 = call <vilib>:"WPI_SwitchGetLimitValue.vi"("error in (no error)"=w1033, "SwitchDevRef"=w1032) -> ("Switch Pressed"=w1024:bool)  [unwired: 7 in, 2 out]
      n273 = Not(x=w1025) -> (.not. x?=w1022:bool)
      n274 = Not(x=w1024) -> (.not. x?=w1023:bool)
      n275 = while {
        tunnel: [0.75 ("Output")] -> w1036
        tunnel: w1029 -> [w1059]
        tunnel: 0.0 ("Output") -> [w1058]
        tunnel: w1027 -> [w1057]
        tunnel: w1026 -> [w1056]
        tunnel: w1023 -> [w1053]
        tunnel: w1022 -> [w1052]
        tunnel: [w1051] -> w1021
        tunnel: w1020 -> [w1050]
        tunnel: w1019 -> [w1049]
        tunnel: w1018 -> [w1048]
        i -> [w1064]
        stop <- w1062 stop-if-true
        n276 = Wait (ms)(milliseconds to wait=u32 100) -> ()  [unwired: 1 out]
        n277 = call <vilib>:"CTRE_Phoenix_MotorControl_Set.vi"("error in (no error)"=w1059, "Output"=w1058, "Control Mode"=w1057, "PhoenixMotorControlDevRef"=w1056) -> ()  [unwired: 6 in, 2 out]
        n278 = call "Drive_Vi.vi"("Middle Thumb"=TRUE, "Y"=-0.5) -> ()  [unwired: 10 in]
        n279 = case shown="False" w1053 {
          tunnel: w1052 -> [_ w1069]
          tunnel: [0.0 ("Output") w1068] -> w1051
          tunnel: [0.0 ("Output") w1067] -> w1047
          frame False {
          }
          frame True {
            n280 = case shown="False" w1069 {
              tunnel: [0.0 ("Output") 0.0 ("Output")] -> w1068
              tunnel: [0.0 ("Output") 0.0 ("Output")] -> w1067
              frame False {
              }
              frame True {
              }
            }
          }
        }
        n281 = call <vilib>:"CTRE_Phoenix_MotorControl_Set.vi"("error in (no error)"=w1050, "Output"=w1047, "Control Mode"=w1049, "PhoenixMotorControlDevRef"=w1048) -> ()  [unwired: 6 in, 2 out]
        n282 = Greater?(x=10, y=w1064) -> (0:w1062:bool)
      }
      n283 = call <vilib>:"CTRE_Phoenix_MotorControl_Set.vi"("error in (no error)"=w1046, "Output"=w1036, "Control Mode"=w1044, "PhoenixMotorControlDevRef"=w1045) -> ()  [unwired: 6 in, 2 out]
      n284 = call <vilib>:"CTRE_Phoenix_MotorControl_Set.vi"("error in (no error)"=w1043, "Output"=w1021, "Control Mode"=w1041, "PhoenixMotorControlDevRef"=w1042) -> ()  [unwired: 6 in, 2 out]
    }
  }
